vi "GUI_Tape_Alignment.vi"() -> ()   [LabVIEW 2020]
uses:
  Shared/GUI_Template/GUI_master/tcp_new_data_event.ctl
  Shared/GUI_Template/GUI_master/tcp new data cluster.ctl
  <vilib>/addons/_JKI.lib/Network_Streams_Connection.llb/NetworkCommand--Cluster.ctl
  <vilib>/addons/_JKI.lib/Network_Streams_Connection.llb/PublicSettings.ctl
  <vilib>/addons/_JKI.lib/Network_Streams_Connection.llb/NetworkConnection.lvclass/NetworkConnection.ctl
  <vilib>/Analysis/NI_AALPro.lvlib
  <vilib>/addons/_JKI.lib/Network_Streams_Connection.llb/NetworkConnection.lvclass
panel:
  out "ZCounts In Range?":bool=TRUE caption="Counts in range for\nz scan?"
  out "Max counts ok align":bool=TRUE
  in  "Min counts for align":dbl=200.0
  in  "Disable pointing correction":bool
  in  "+- from current":dbl=0.7 format="%#_13g"
  in  "set limits":bool caption="set limits basd on current position"
  in  "wangle upper limit":dbl=0.5682929999999999
  in  "wangle lower limit":dbl=-0.831707
  in  "vangle lower limit":dbl=-0.8982979999999999
  in  "vangle upper limit":dbl=0.501702
  out "move In Range W":bool=TRUE
  out "move In Range V":bool=TRUE
  in  "position::3":dbl=-3.999987 caption="vert stage pos" min=-48.0 max=0.0 step=0.01 format="%.5f"
  in  "GUIdevice 3":string="STAGE-PL1-Vertical"
  in  "Check beam quality":bool
  in  "Zpos Scan":bool
  in  "2ndmomW0y::1":dbl=55.508877 caption="w0 Y" min=0.0 max=999999.0
  in  "MaxCounts::1":dbl=1624.0 caption="Max Counts" min=0.0 max=999999999.0
  in  "xyzuvw::2":string="4.700098E+0,4.999902E+0,-1.803888E-7,1.749400E-6,-6.503994E-1,9.120211E-2" caption="Hex position"
  out "slow response":string="HEX-PL1-3-Small>>setxyzuvw>>4.700083,4.999904,0.000001,0.000007,-0.650383,0.091191>>no error,"
  in  "tab":T1(tab)=enum."Controls"
  out "Zpos and w0 Y":dbl(graph)=-4.0
  out "Alignment attempts":i32=3
  out "Waveform Chart 2":u32(graph)=298
  out "Movement time":u32=298
  out "Alignment time":u32=4006
  out "Waveform Chart 3":u32(graph)=4006
  out "Waveform Chart 4":i32(graph)=3
  out "Waveform Chart":cluster{"centroidx::1":dbl, "centroidy::1":dbl}(graph)={"centroidx::1"=1170.062134, "centroidy::1"=572.23645}
  out "Zpos and w0 Y 2":dbl(graph)=3261.0
  out "X Graph":T2(graph)
  out "Y Graph":T3(graph)
  out "X slope":dbl
  out "Y slope":dbl
  out "Y error":dbl
  out "X error":dbl
  in  "Calibration steps":dbl=8.0
  in  "Calibration Angle":cluster{"X":dbl, "Y":dbl}={"X"=0.01, "Y"=0.01}
  in  "Export":bool caption="Export calibration"
  in  "Import":bool caption="Import calibration"
  in  "Dont z scan if above this counts":dbl=2000.0
  in  "Central position of z scan":dbl=-4.0
  in  "Diagnostic type":enum16{"Max counts", "w0 Y"}(ring)
  in  "Disable Zpos Scan":bool=TRUE
  in  "zpos scan increment":dbl=1.0
  in  "zpos scan range":dbl=6.0
  in  "Newmark for vertical":bool=TRUE
  in  "Min counts for z scan":dbl=20.0
  in  "central z upper limit":dbl=-6.0
  in  "central z lower limit":dbl=-6.0
  in  "always z scan":bool
  in  "Buffer":dbl=0.9 format="%#_13g"
  in  "Accuracy limit":cluster{"X":dbl, "Y":dbl}={"X"=5.0, "Y"=5.0}
  out "Connected?":bool=TRUE
  in  "Aligned message":T4={"Command"="Alignment Done!", "Arguments"=variant(string "Arguments are variants. Wire anything!"), " Msg Id"=0}
  in  "Settings":T5={"My Name"="AlignmentGUI", "Remote IP Address"="", "Remote Name"="TapeDrive"}
  out "Public Settings":T5={"My Name"="AlignmentGUI", "Remote IP Address"="", "Remote Name"="TapeDrive"}
  out "Message count":i32=306
  out "Incoming Messages":T4[](array[typedef])=[{"Command"="ping", "Arguments"=variant, " Msg Id"=0}]
  out "Connected? 2":bool=TRUE
  in  "Stop z scan":bool
  out "Max vs z":T6(graph)={"Hexapod zscan positions"=[-9.0, -8.0, -7.0, -6.0, -5.0, -4.0, -3.0], "Hexapod zscan diagnostic"=[227.0, 362.0, 861.0, 1607.0, 1974.0, 3261.0, 1052.0]}
  out "msg":string="Macro: Alignment"
  out "tcp data event":T7
  in  "Target.Y::1":dbl=571.0 caption="Target Y" min=0.0 max=2000.0
  in  "Target.X::1":dbl=1173.0 caption="Target X" min=0.0 max=2000.0
  in  "Stop":bool
  out "Remaining States":string
  out "Current State":string="Exit"
  in  "Calibrate":bool
  in  "wangle::2":dbl=0.091202 caption="W" min=-1.0 max=1.0 step=0.01 format="%.5f"
  in  "vangle::2":dbl=-0.650399 caption="V" min=-1.0 max=1.0 step=0.01 format="%.5f"
  in  "centroidy::1":dbl=590.313232 caption="Centroid Y" min=0.0 max=0.0
  in  "centroidx::1":dbl=1182.786255 caption="Centroid X" min=0.0 max=0.0
  in  "ypos::2":dbl=4.999902 caption="Y" min=-10.0 max=10.0 step=0.01 format="%.5f"
  in  "xpos::2":dbl=4.700098 caption="X" min=-10.0 max=10.0 step=0.01 format="%.5f"
  in  "zpos::2":dbl=-0.0 caption="Z" min=-5.0 max=5.0 step=0.01 format="%.5f"
  in  "uangle::2":dbl=2e-06 caption="U" min=-1.0 max=1.0 step=0.01 format="%.5f"
  out "error IO 2":errorcluster
  in  "GUIdevice 2":string="HEX-PL1-3-Small"
  in  "GUIdevice 1":string="CAM-PL1-TapeDrivePointing"
  in  "Align Tape":bool
  # "Tape drive device cmd to align"
  # "Action: Get Beam Diagnostic>> Check Quality"
  # "disabled or counts high enough"
  # "If enabled. z scan only if max counts too low"
  # "Macro: Alignment"
  # "Macro: Hexapod Zpos Scan\nMacro: Alignment"
  # "Loop of\nAction: Move>> Zpos Scan\nAction: Get Beam Diagnostic>>Zpos Scan\n\nThen \n\nAction: Find Best Zpos"
  # "Align Tape button"
  # "Macro: Alignment"
  # "Action: Find Best Zpos\n#which calls\nAction: Move>> Best Zpos\nMacro: Alignment\n#does aligment get called twice?"
  # "Counts too low or disabled"
  # "If enabled and sufficient counts"
  # "Do nothing"
  # "Update: Alignment Constants\nAction: Get Centroid>> Align"
  # "If aligned or  align disabled"
  # "Action: Move>> Align\nAction: Get Centroid>> Align"
  # "Action: Send Response"
  # "Note: If action move tries too many times, it empties state machine and tape drive never gets a response"
  # "Align"
  # "Z scan"
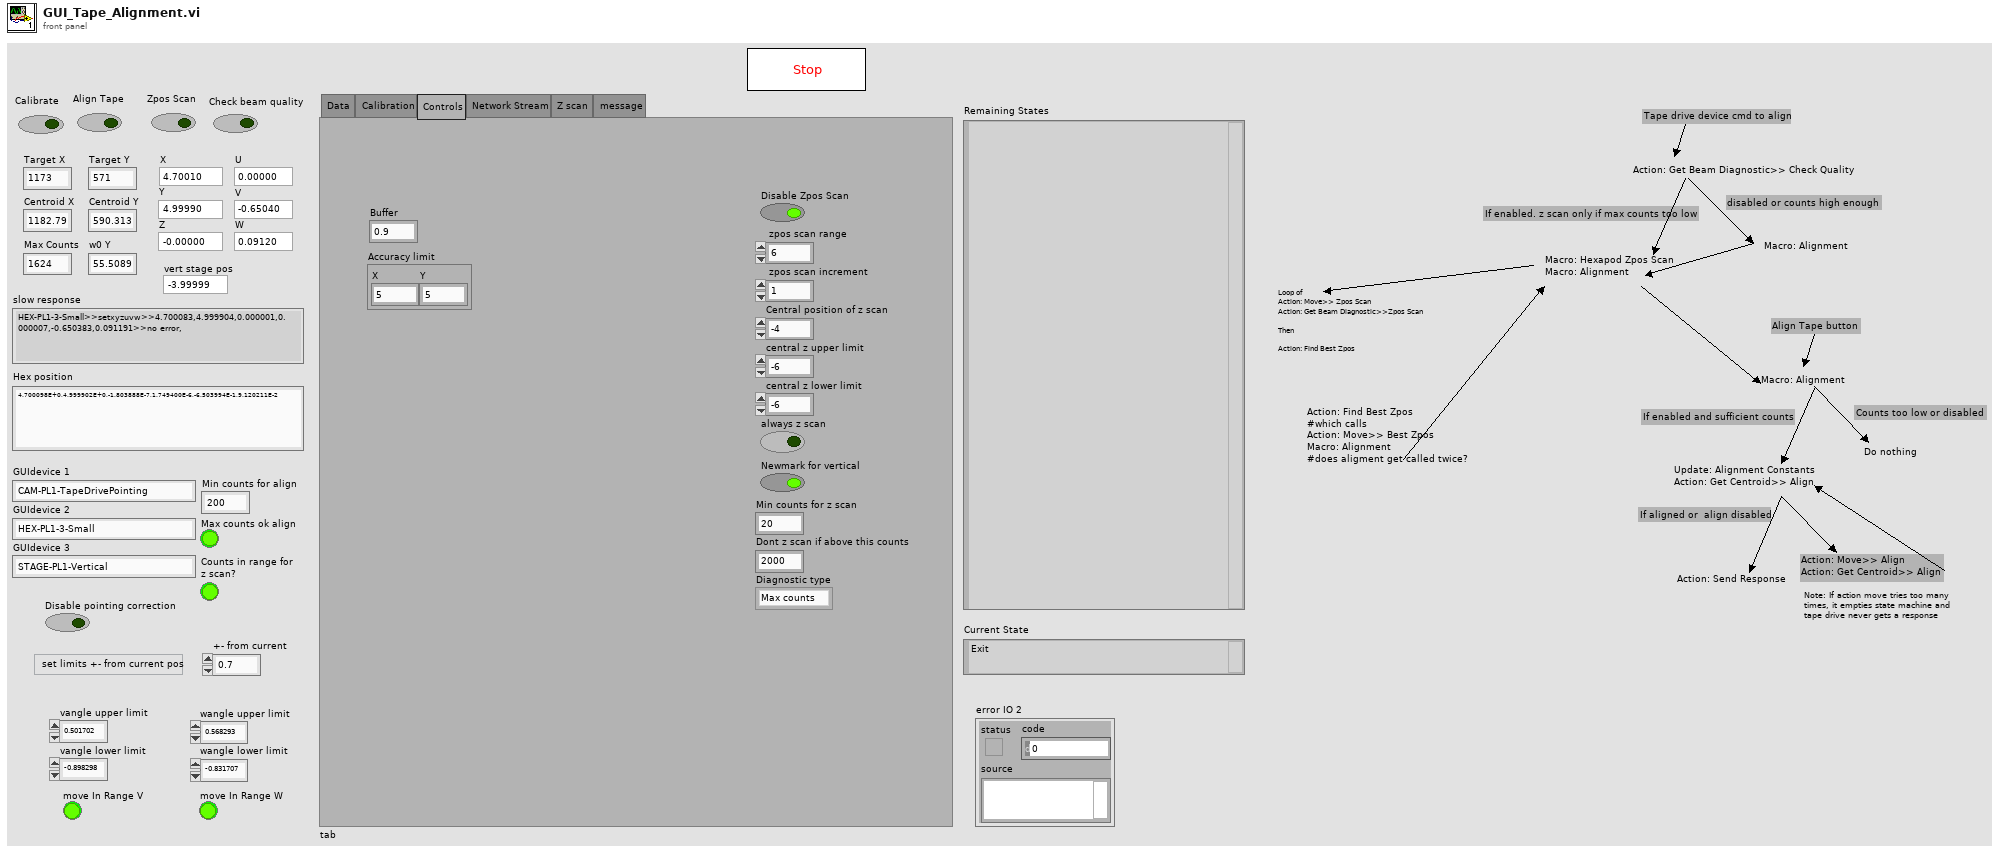
[diagram p1: front panel]
types:
  T1 = enum32{"Data", "Calibration", "Controls", "Network Stream", "Z scan", "message"}
  T2 = cluster{"Centroids.x":dbl[], "Best Linear Fit":dbl[]}[]
  T3 = cluster{"Centroids.y":dbl[], "Best Linear Fit":dbl[]}[]
  T4 = typedef "NetworkConnection.lvclass/NetworkCommand--Cluster.ctl" = cluster{"Command":string, "Arguments":variant, " Msg Id":i32}
  T5 = typedef "NetworkConnection.lvclass/PublicSettings.ctl" = cluster{"My Name":string, "Remote IP Address":string, "Remote Name":string}
  T6 = cluster{"Hexapod zscan positions":dbl[], "Hexapod zscan diagnostic":dbl[]}
  T7 = typedef "tcp_new_data_event.ctl" = refnum<user-event>
  T8 = typedef "tcp new data cluster.ctl" = cluster{"EventEnum":enum16{"new data", "connection status update"}, "Device name":string}
  T9 = enum32{"Data", "Calibration", "Controls", "Network Stream", "Z scan"}
  T10 = enum32{"Invalid", "Standard", "Closed", "Hidden", "Minimized", "Maximized"}
  T11 = enum32{"invalid app kind", "Development System", "Run Time System", "Student Edition", "Embedded LabVIEW", "Evaluation", "Custom"}
  T12 = cluster{"Messages[0]":T4, "Messages[1]":T4, "Messages[2]":T4, "Messages[3]":T4, "Messages[4]":T4, "Messages[5]":T4, "Messages[6]":T4, "Messages[7]":T4, "Messages[8]":T4}
  T13 = cluster{"Core":cluster{"Current VI Reference":refnum<vi>, "Close Panel on Exit?":bool}, "Difference":cluster{"X":dbl, "Y":dbl}, "Scale Factor":cluster{"X":dbl, "Y":dbl}, "Centroids":cluster{"Centroids.x":dbl[], "Centroids.y":dbl[]}, "Calibration Angle ":cluster{"X":dbl, "Y":dbl}, "Accuracy limit":cluster{"X":dbl, "Y":dbl}, "Calibration steps":dbl, "NetworkConnection out":refnum<class "NetworkConnection.lvclass">, "Messages":i32, "Alignment attempts":i32, "Timer":cluster{"T1":i32, "T2":i32}, "Hexapod positions":cluster{"P1":string, "P2":string}, "Beam diagnostic cutoffs":cluster{"MaxCounts":dbl, "w0 Y":dbl}, "Hexapod zscan data":cluster{"Hexapod zscan positions":dbl[], "Hexapod zscan diagnostic":dbl[], "Index":i32, "Best Zpos":dbl}, "Diagnostic type":string}
  T14 = cluster{"Hexapod zscan positions":dbl[], "Hexapod zscan diagnostic":dbl[], "Index":i32, "Best Zpos":dbl}
  T15 = cluster{"Centroids.x":dbl[], "Centroids.y":dbl[]}
  T16 = cluster{"Current VI Reference":refnum<vi>, "Close Panel on Exit?":bool}
  T17 = cluster{"Centroids.x":dbl[], "Best Linear Fit":dbl[]}
  T18 = cluster{"Centroids.y":dbl[], "Best Linear Fit":dbl[]}
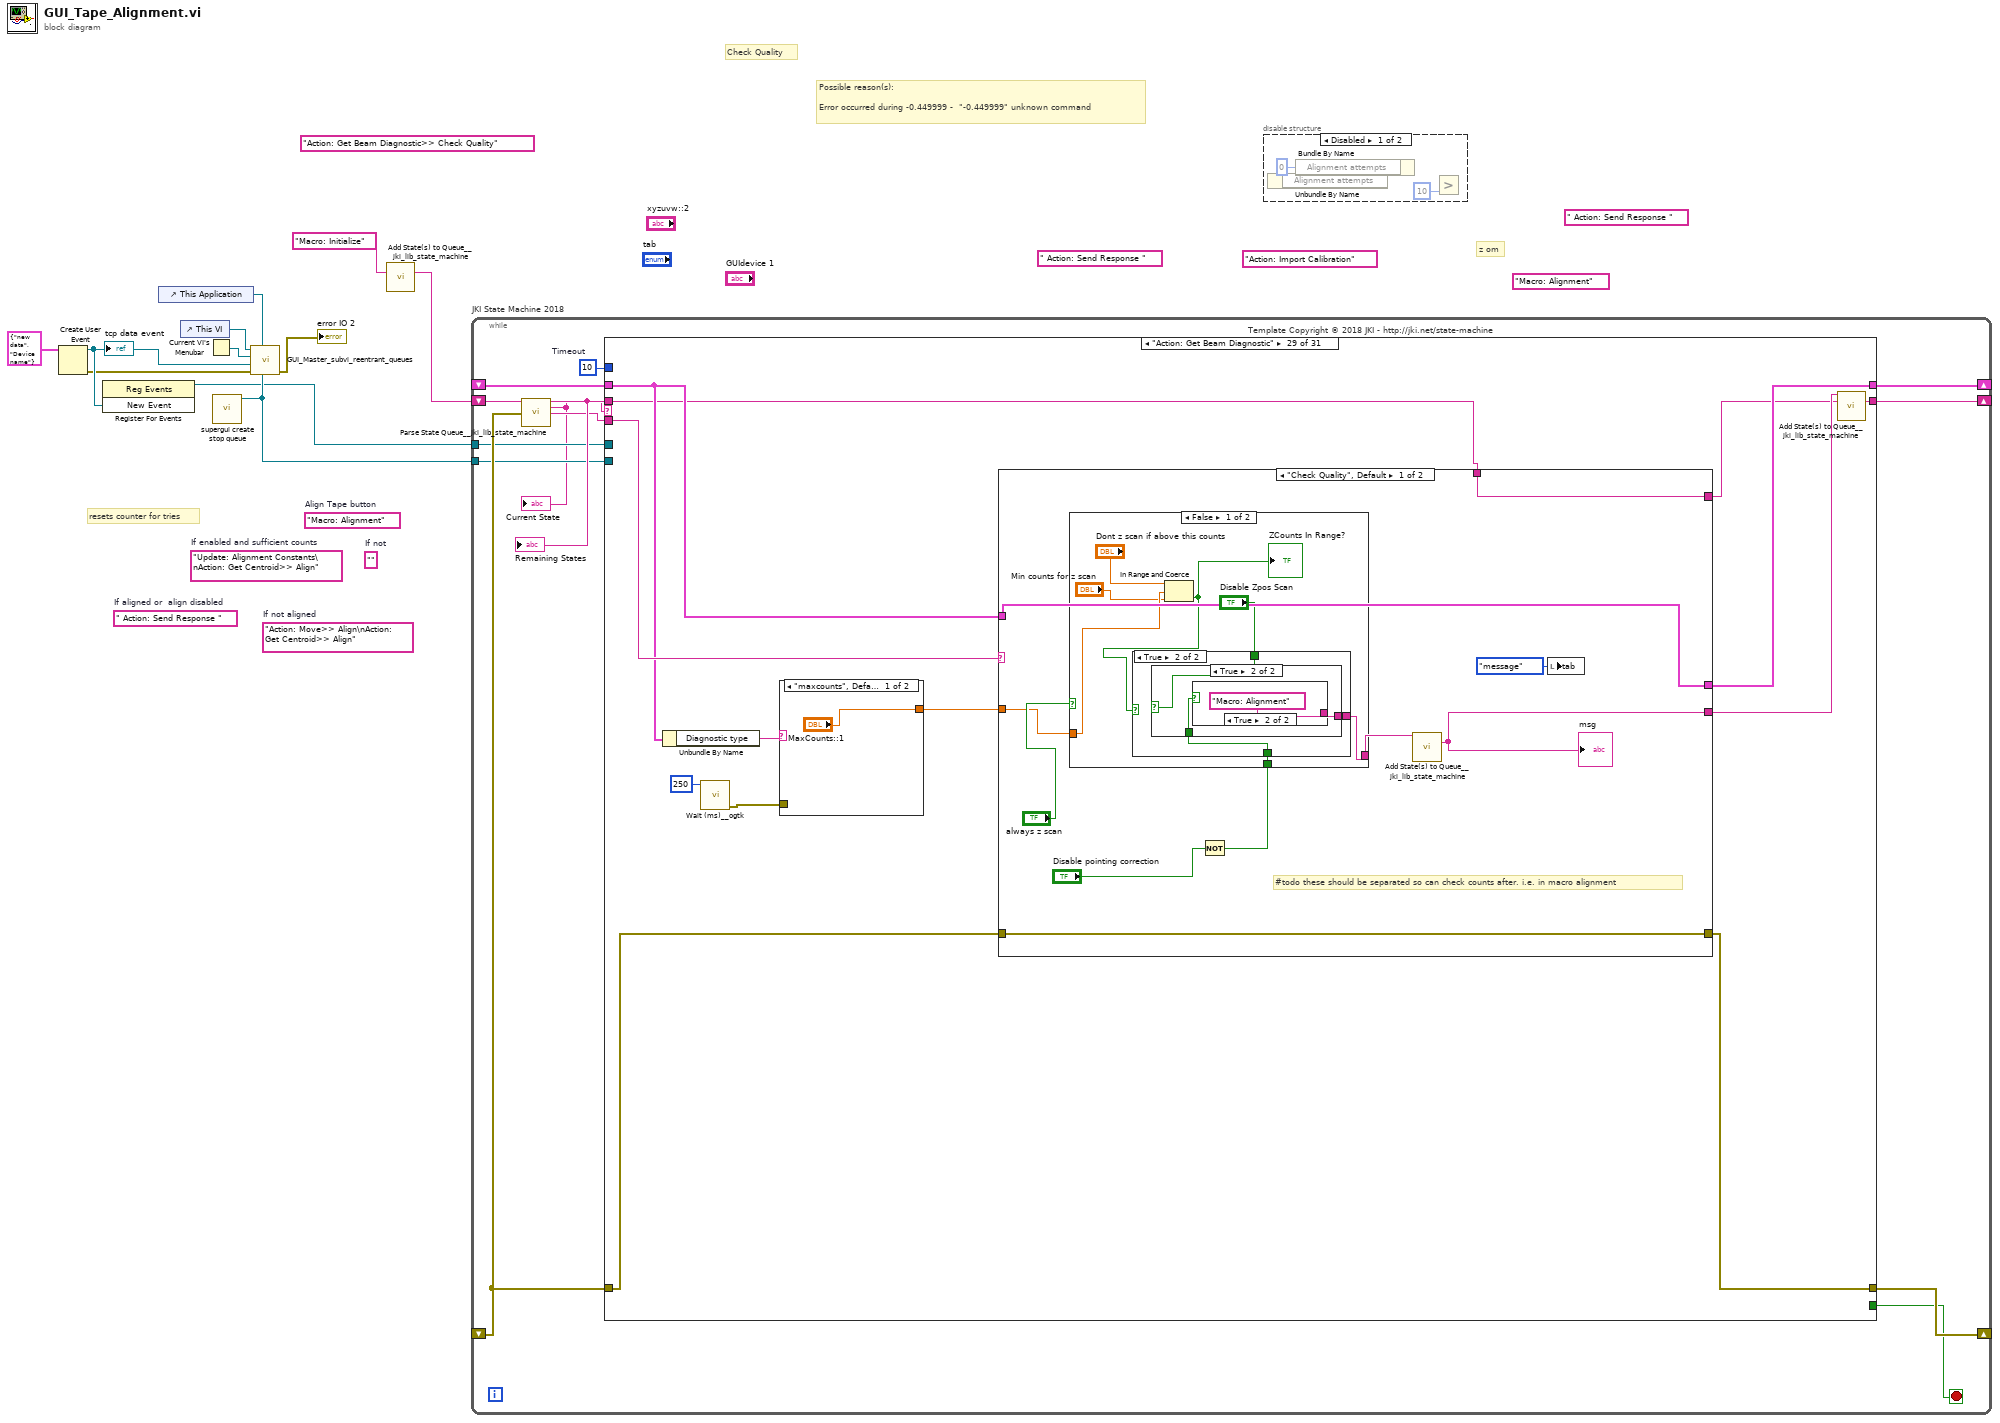
[diagram p0: block diagram]
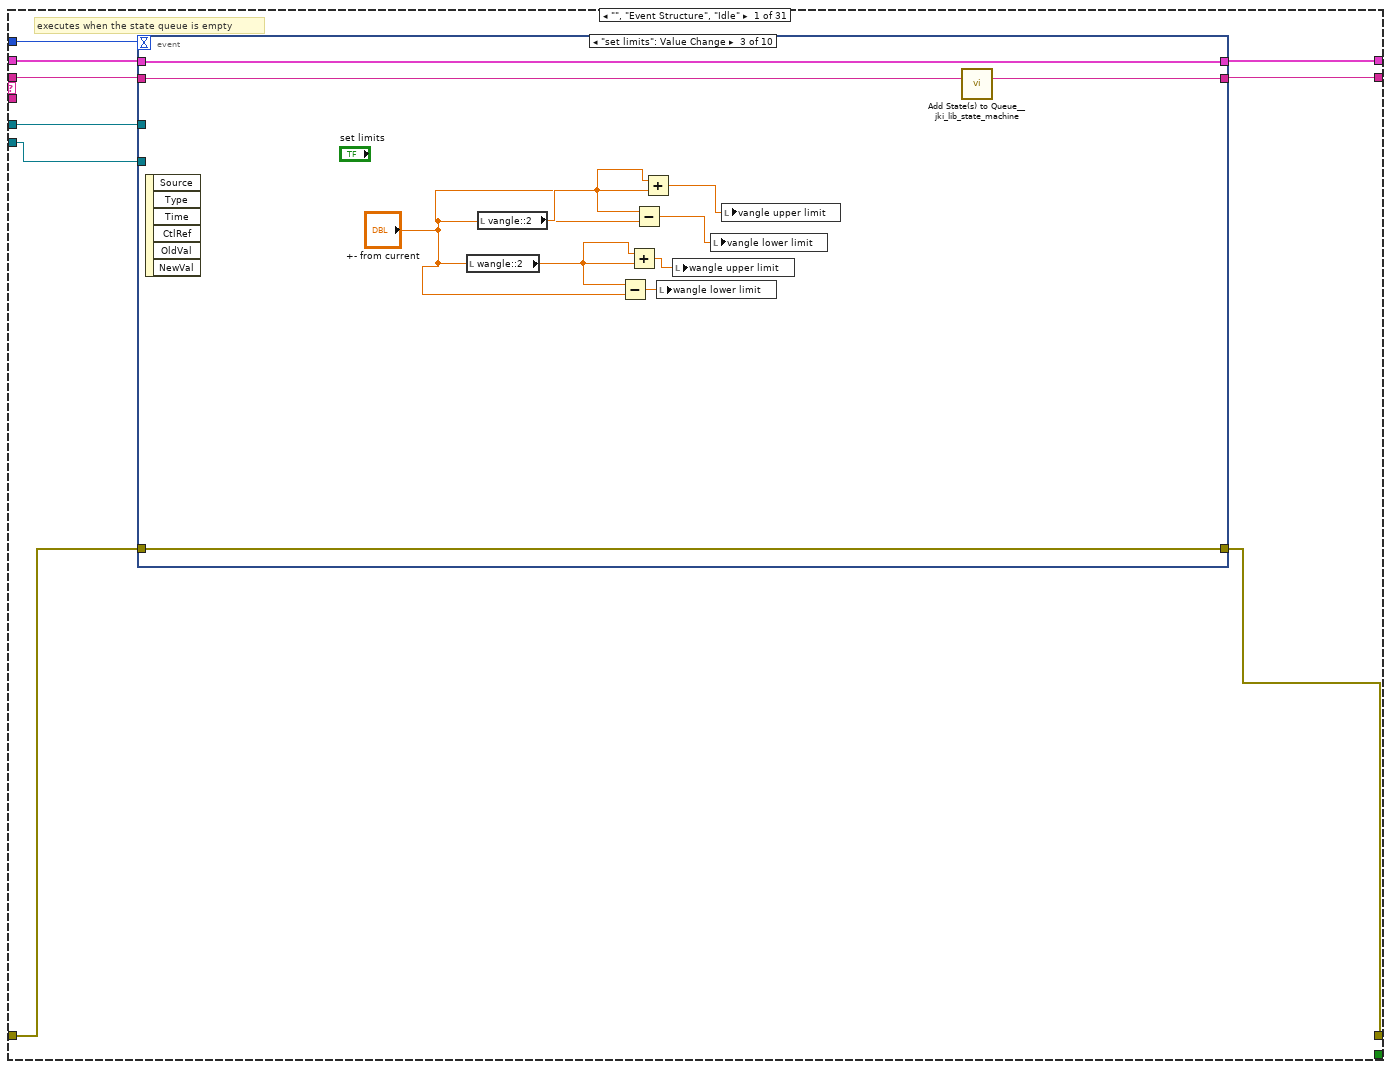
[diagram p3: hidden frame]
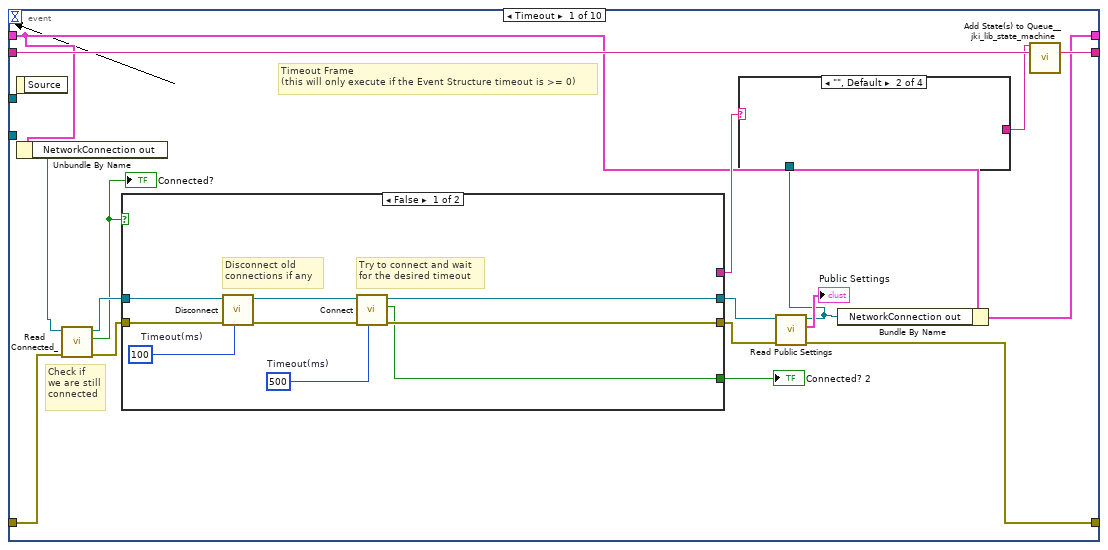
[diagram p4: hidden frame]
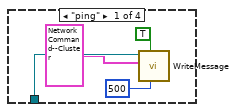
[diagram p5: hidden frame]
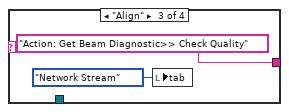
[diagram p6: hidden frame]
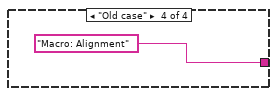
[diagram p7: hidden frame]
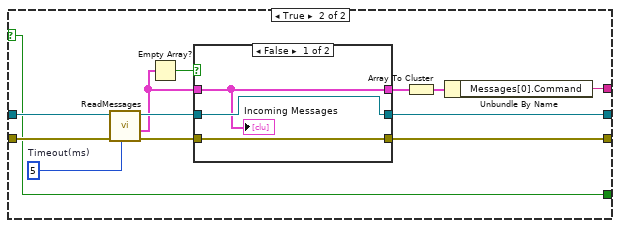
[diagram p8: hidden frame]
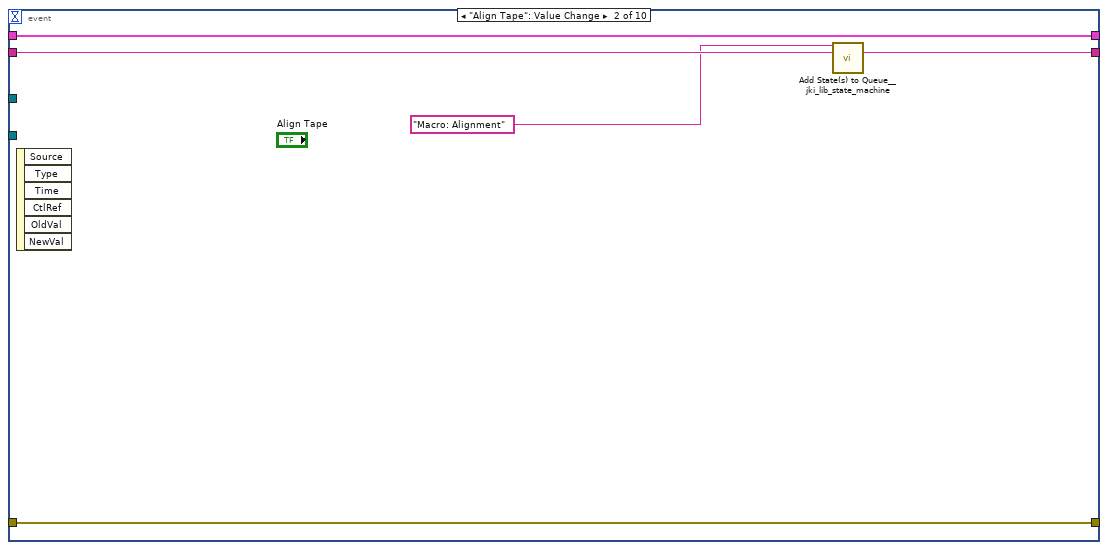
[diagram p10: hidden frame]
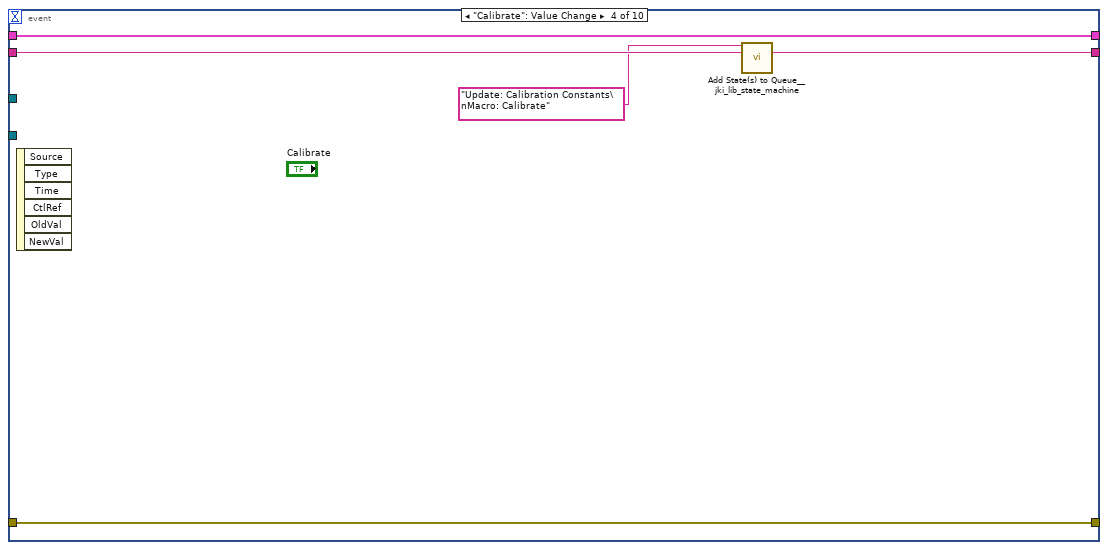
[diagram p11: hidden frame]
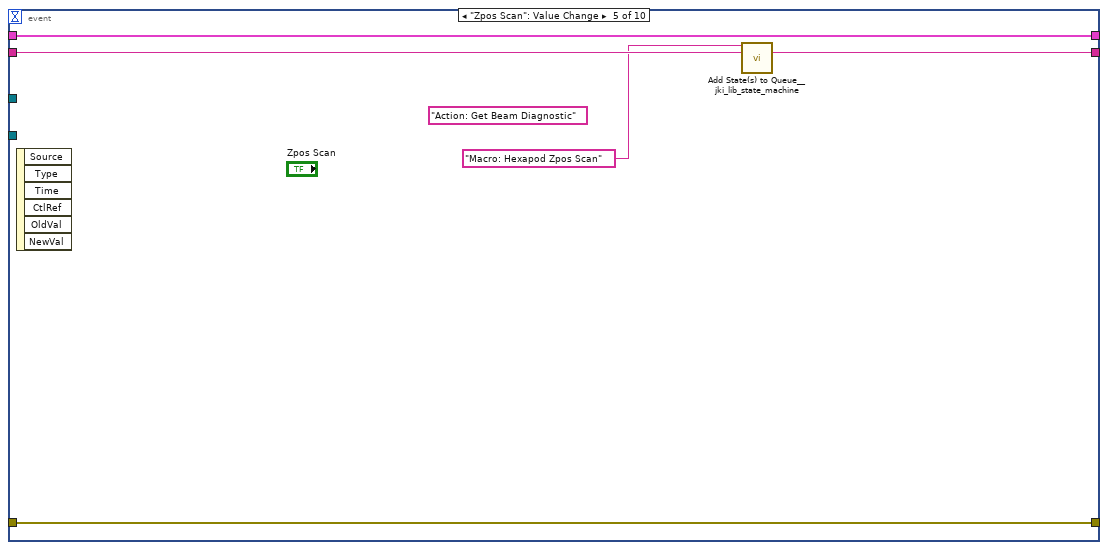
[diagram p12: hidden frame]
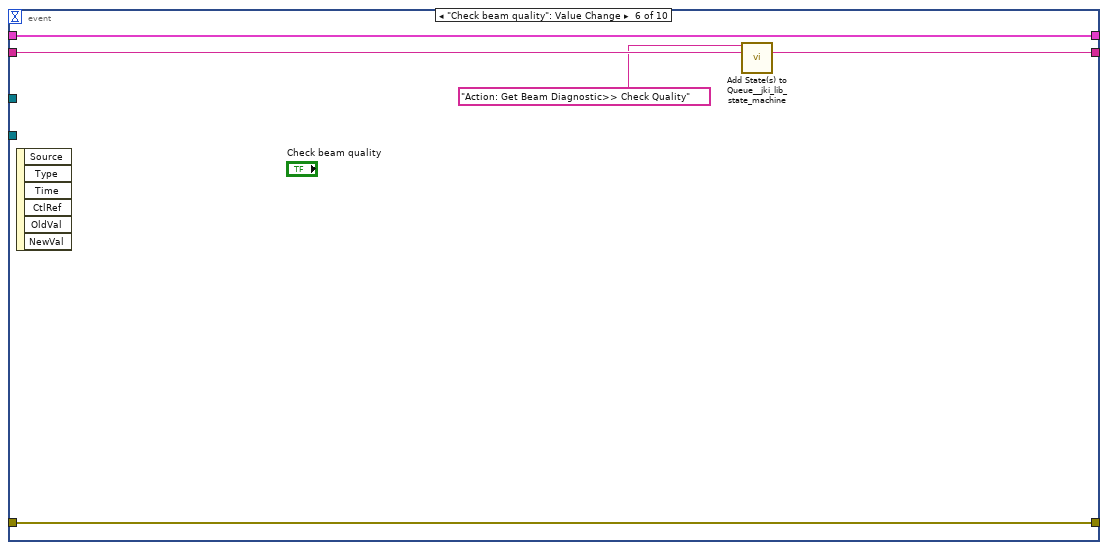
[diagram p13: hidden frame]
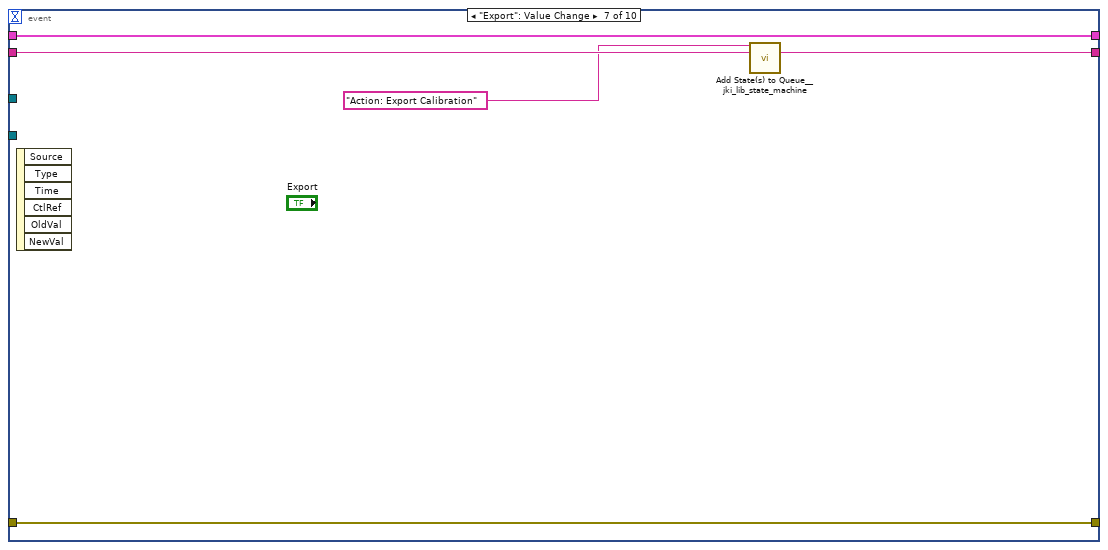
[diagram p14: hidden frame]
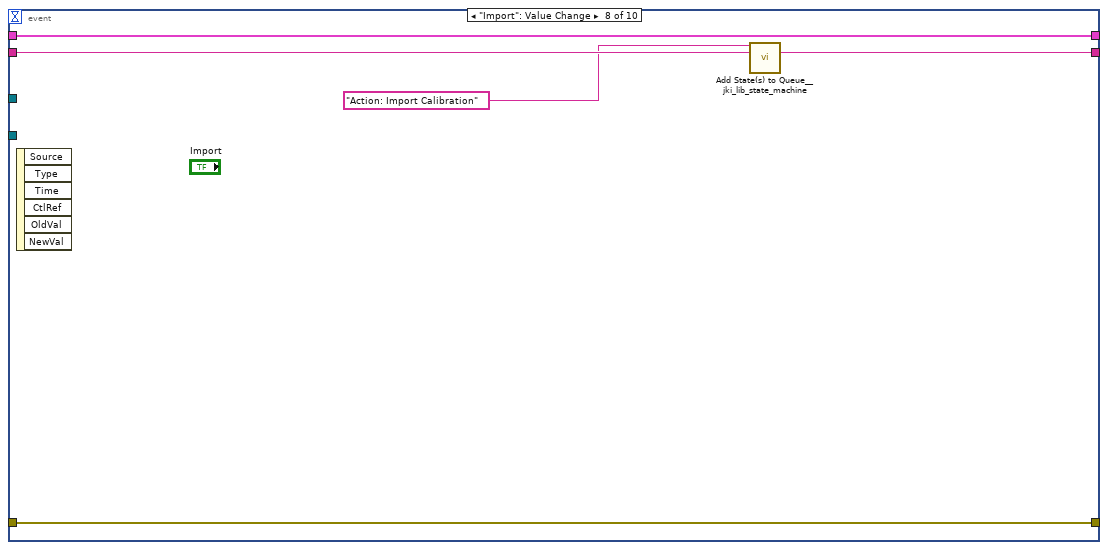
[diagram p15: hidden frame]
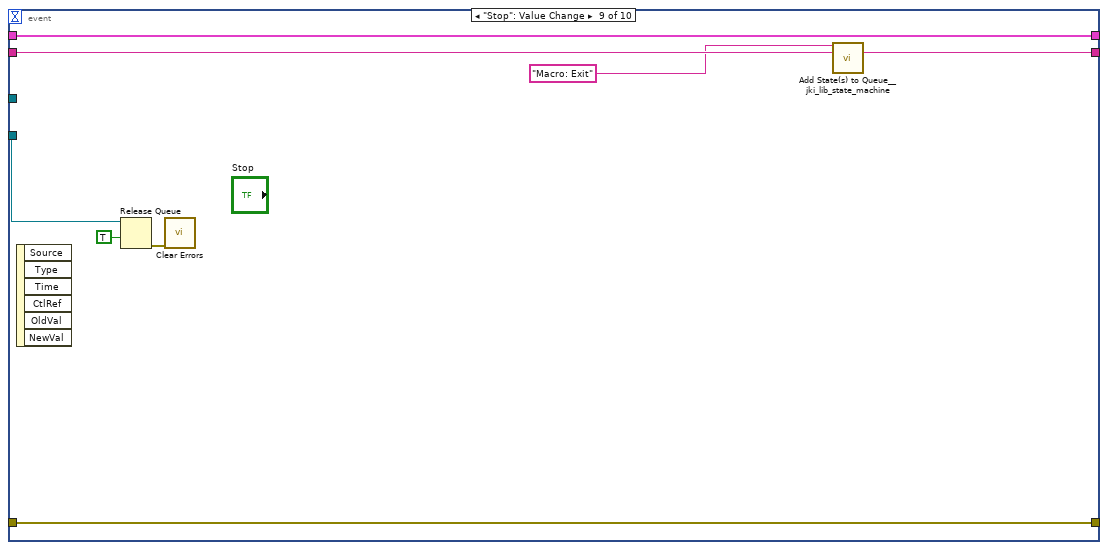
[diagram p16: hidden frame]
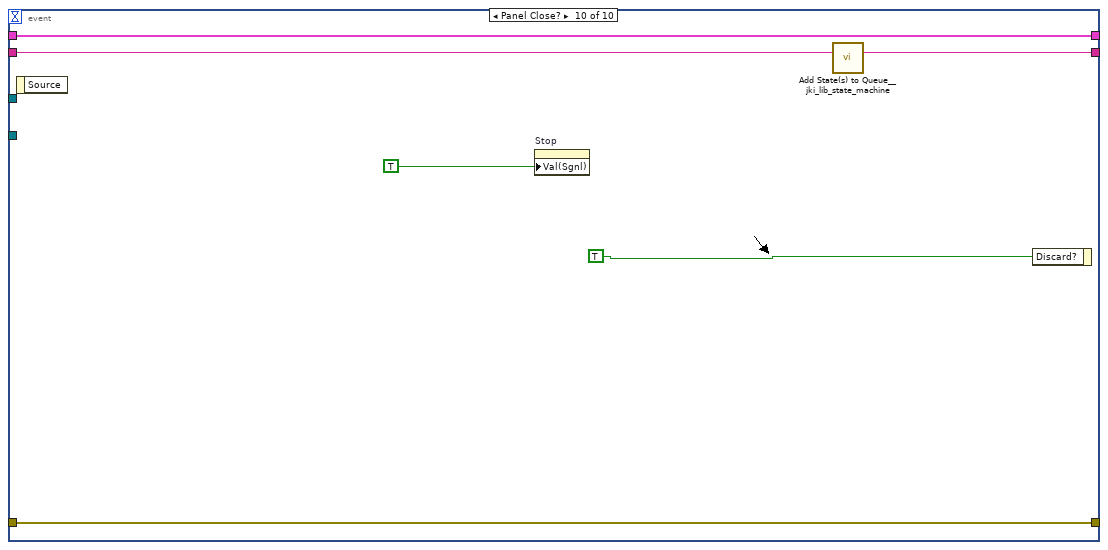
[diagram p17: hidden frame]
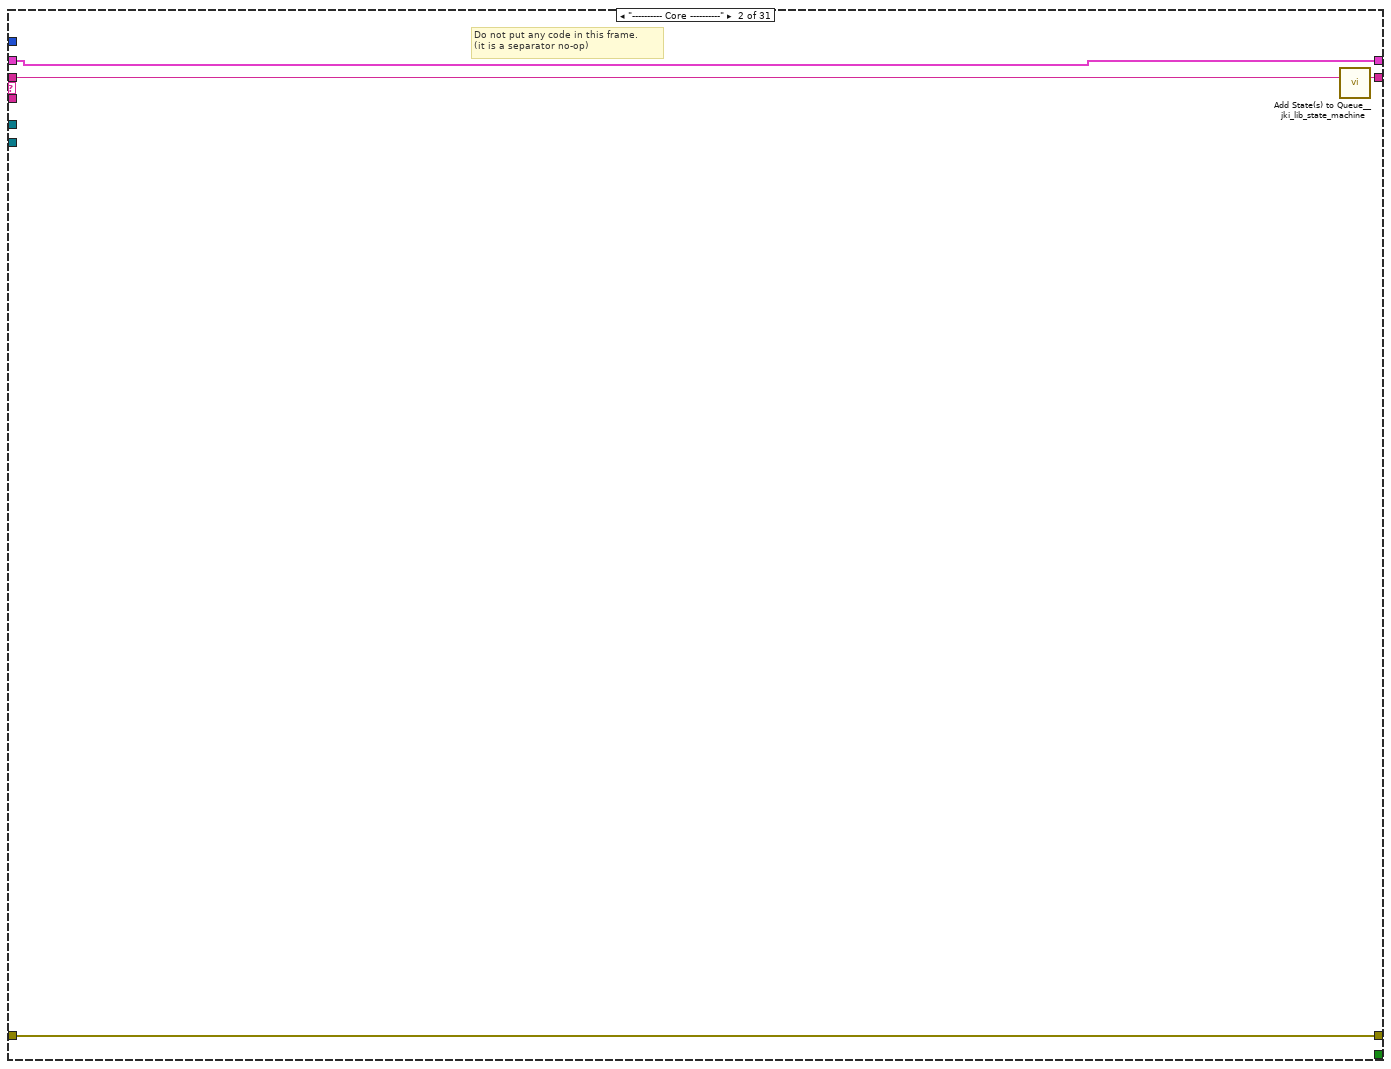
[diagram p18: hidden frame]
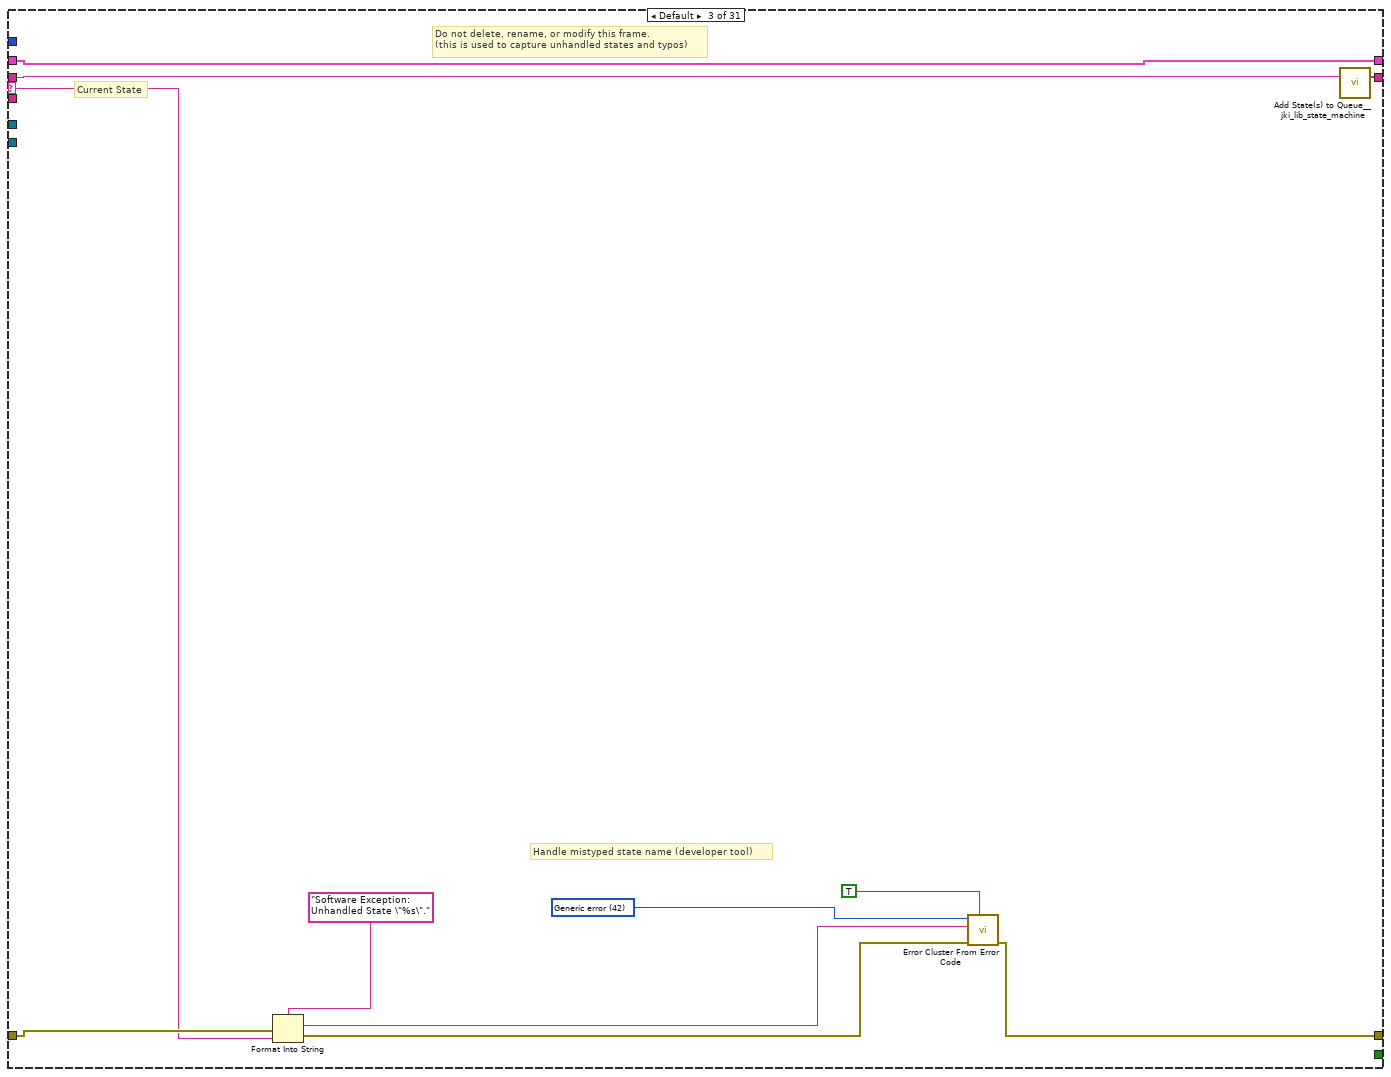
[diagram p19: hidden frame]
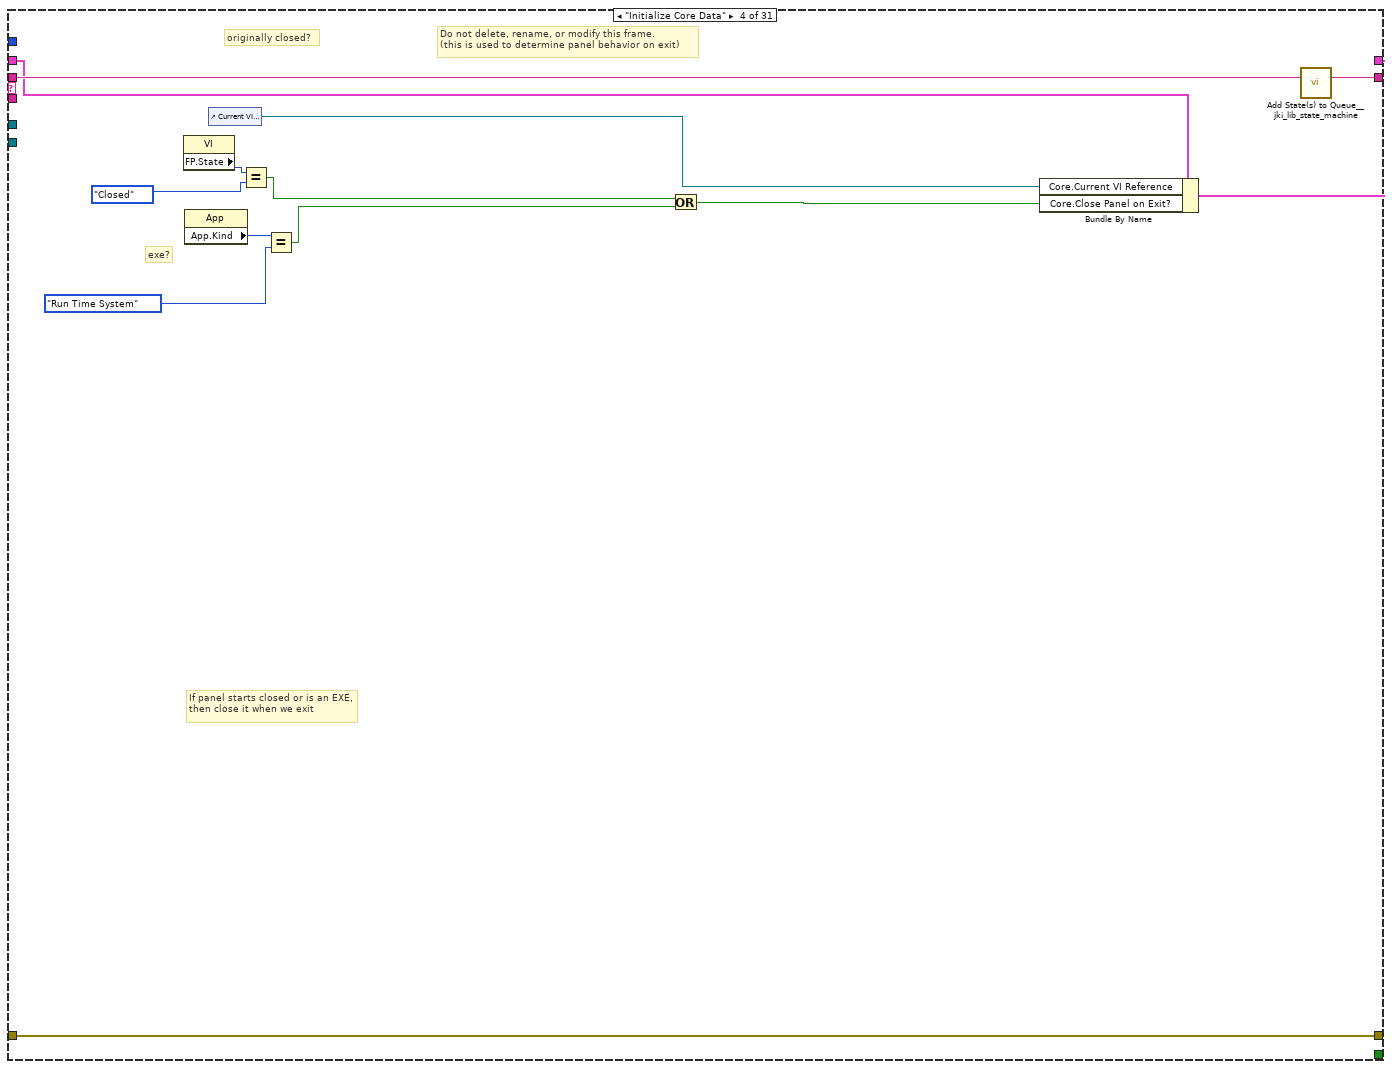
[diagram p20: hidden frame]
diagram:
  (unwired) " Action: Send Response "
  (unwired) "Action: Get Beam Diagnostic>> Check Quality"
  (unwired) "Action: Move>> Align\nAction: Get Centroid>> Align"  # If not aligned
  (unwired) " Action: Send Response "  # If aligned or  align disabled
  (unwired) ""  # If not
  (unwired) "Update: Alignment Constants\nAction: Get Centroid>> Align"  # If enabled and sufficient counts
  (unwired) "Macro: Alignment"  # Align Tape button
  (unwired) " Action: Send Response "
  (unwired) "Action: Import Calibration"
  (unwired) "Macro: Alignment"
  # "resets counter for tries"
  # "z om"
  # "Check Quality"
  # "Possible reason(s):\n\nError occurred during -0.449999 -  \"-0.449999\" unknown command"
  n1 = Create User Event(user event datatype=T8 {"EventEnum"=enum."new data", "Device name"="Device name"} ("New Event")) -> (user event=w8:refnum<user-event>, error out=w7:errorcluster)  [unwired: 1 in]
  "tcp data event" <- w8
  n2 = register-events(w8) -> (reference out=w1:refnum<event-registration>)  [unwired: 2 in, 1 out]
  n3 = control-ref of="This Application"() -> (w9:refnum<vi>)
  n4 = control-ref of="This VI"() -> (w4:refnum<vi>)
  n5 = Current VI's Menubar() -> (w5:refnum<k9>)
  n6 = call "supergui create stop queue.vi"() -> ("STOP Queue out"=w2:refnum<queue>)  [unwired: 11 in]
  n7 = call "GUI_Master_subvi_reentrant_queues.vi"("STOP Queue in"=w2, "This Application"=w9, "error in (no error)"=w7, "tcp data event"=w8, "Caller menu reference"=w5, "Caller VI ref"=w4) -> ("error out"=→"error IO 2":errorcluster)  [unwired: 5 in]
  n8 = call <vilib>:"Add State(s) to Queue__jki_lib_state_machine.vi"("State(s) in (\"\")"="Macro: Initialize") -> ("States Out"=w11:string)  [unwired: 14 in]
  n9 = while "JKI State Machine 2018" {
    shift-right: [w19] -> _
    shift-left: _ -> [w18]
    shift-right: [w21] -> _
    shift-left: _ -> [w16]
    shift-right: [w20] -> _
    shift-left: w11 -> [w22]
    tunnel: w1 -> [w15]
    tunnel: w2 -> [w14]
    stop <- w13 stop-if-true
    w17 = 10  # Timeout
    # "Template Copyright © 2018 JKI - http://jki.net/state-machine"
    n10 = call <vilib>:"Parse State Queue__jki_lib_state_machine.vi"("State Queue"=w22, "Error In (no error)"=w16) -> ("Remaining States"=w24:string, "Current State"=w12:string, "Arguments"=w23:string)  [unwired: 11 in]
    "Current State" <- w12
    "Remaining States" <- w24
    n11 = case shown="\"Action: Get Beam Diagnostic\"" w12 {
      selector: w12 -> [_ _ w145 _ _ _ _ _ _ _ _ _ _ _ _ _ _ _ _ _ _ _ _ _ _ _ _ _ _ _ _]
      tunnel: w24 -> [w33 w144 w149 w168 w174 w179 w183 w203 w211 w215 w219 w225 w236 w305 w310 w320 w339 w372 w394 w401 w407 w415 w420 w434 w477 w659 w667 w678 w680 w755 w779]
      tunnel: w23 -> [_ _ _ _ _ _ _ _ _ _ _ w220 w230 _ _ _ _ _ _ _ _ _ _ w424 w476 _ _ _ w690 _ _]
      tunnel: w18 -> [w31 w141 w147 w161 w171 w177 w180 _ w207 w212 w217 w223 w232 w302 w307 w313 w343 w368 w391 w398 w405 w414 w417 w425 w502 w655 w665 w673 w684 w752 w772]
      tunnel: [w30 w142 w151 w165 errorcluster {"status"=FALSE, "code"=0, "source"=""} ("error out") w176 w181 w200 w204 w213 w216 w221 w233 w303 w308 w322 w351 w373 w392 w399 w408 w410 w418 w426 w495 w657 w661 w668 w685 w753 w766] -> w21
      tunnel: w16 -> [w29 w142 w150 w165 w170 w176 w181 w200 w208 w213 w216 w222 w234 w303 w308 w322 w351 w373 w392 w399 w408 w410 w418 w423 w501 w657 w662 w669 w686 w753 w776]
      tunnel: [w32 w143 w148 w167 w173 w178 w182 w202 w210 w214 w218 w224 w235 w304 w309 w323 w352 w374 w393 w400 w409 w416 w419 w433 w503 w658 w666 w677 w691 w754 w778] -> w20
      tunnel: [_ _ _ _ _ TRUE _ _ _ _ _ _ _ _ _ _ _ _ _ _ _ _ _ _ _ _ _ _ _ _ _] -> w13
      tunnel: [w28 w141 w147 w166 w171 w177 w180 w201 w207 w212 w217 w223 w232 w302 w307 w311 w342 w369 w391 w398 w404 w413 w417 w432 w481 w656 w665 w676 w687 w751 w773] -> w19
      tunnel: w17 -> [w27 _ _ _ _ _ _ _ _ _ _ _ _ _ _ _ _ _ _ _ _ _ _ _ _ _ _ _ _ _ _]
      tunnel: w15 -> [w26 _ _ _ _ _ _ _ _ _ _ _ _ _ _ _ _ _ _ _ _ _ _ _ _ _ _ _ _ _ _]
      tunnel: w14 -> [w25 _ _ _ _ _ _ _ _ _ _ _ _ _ _ _ _ _ _ _ _ _ _ _ _ _ _ _ _ _ _]
      frame "", "Event Structure", "Idle" {
        # "executes when the state queue is empty"
        n12 = event shown="[2] \"set limits\": Value Change" {
          selector: _ -> [_ _ _ _ _ _ _ _ _ _]
          dyn-events: _ -> [_ _ _ _ _ _ _ _ _ _]
          timeout: w27 -> [_ _ _ _ _ _ _ _ _ _]
          tunnel: w33 -> [w50 w90 w101 w105 w110 w115 w119 w124 w134 w140]
          tunnel: [w49 w89 w100 w103 w109 w113 w120 w125 w133 w139] -> w32
          tunnel: w31 -> [w40 w86 w98 w106 w111 w116 w121 w126 w131 w137]
          tunnel: [w37 w88 w99 w102 w108 w112 w117 w122 w132 w138] -> w30
          tunnel: w29 -> [w45 w88 w99 w102 w108 w112 w117 w122 w132 w138]
          tunnel: [w41 w86 w98 w106 w111 w116 w121 w126 w131 w137] -> w28
          tunnel: w26 -> [_ _ _ _ _ _ _ _ _ _]
          tunnel: w25 -> [_ _ _ _ _ _ _ _ w127 _]
          event Timeout {
            # "Check if\nwe are still\nconnected"
            # "Timeout Frame\n(this will only execute if the Event Structure timeout is >= 0)"
            n13 = event-data() -> ()  [unwired: 1 in, 1 out]
            n14 = Unbundle By Name(w40) -> ("NetworkConnection out"=w42:refnum<class "NetworkConnection.lvclass">)
            n15 = call <vilib>:"Read Connected_.vi"("error in (no error)"=w45, "NetworkConnection in"=w42) -> ("error out"=w48:errorcluster, "Connected?"=w46:bool, "NetworkConnection out"=w47:refnum<class "NetworkConnection.lvclass">)  [unwired: 7 in]
            "Connected?" <- w46
            n16 = case shown="False" w46 {
              selector: w46 -> [_ w67]
              tunnel: w48 -> [w62 w77]
              tunnel: w47 -> [w64 w78]
              tunnel: [w65 w72] -> w39
              tunnel: [w66 w71] -> w38
              tunnel: [_ w75] -> w44
              tunnel: [w58 w67] -> w35
              frame False {
                w59 = 500  # Timeout(ms)
                w60 = 100  # Timeout(ms)
                # "Try to connect and wait\nfor the desired timeout"
                # "Disconnect old\nconnections if any"
                n17 = call <vilib>:"Disconnect.vi"("Timeout ms (1000)"=w60, "error in (no error)"=w62, "NetworkConnection in"=w64) -> ("error out"=w61:errorcluster, "NetworkConnection out"=w63:refnum<class "NetworkConnection.lvclass">)  [unwired: 7 in]
                n18 = call <vilib>:"Connect.vi"("Timeout(ms)"=w59, "error in (no error)"=w61, "NetworkConnection in"=w63) -> ("error out"=w66:errorcluster, "Connected?"=w58:bool, "NetworkConnection out"=w65:refnum<class "NetworkConnection.lvclass">)  [unwired: 6 in]
              }
              frame True {
                w79 = 5  # Timeout(ms)
                n19 = call <vilib>:"ReadMessages.vi"("Timeout(ms)"=w79, "error in (no error)"=w77, "NetworkConnection in"=w78) -> ("error out"=w70:errorcluster, "Messages"=w68:T4[], "NetworkConnection out"=w73:refnum<class "NetworkConnection.lvclass">)  [unwired: 4 in, 2 out]
                n20 = Empty Array?(array=w68) -> (empty?=w74:bool)
                n21 = case shown="False" w74 {
                  tunnel: w73 -> [w82 w85]
                  tunnel: [w82 w85] -> w72
                  tunnel: [w81 w84] -> w71
                  tunnel: w70 -> [w81 w84]
                  tunnel: [w80 w83] -> w69
                  tunnel: w68 -> [w80 w83]
                  frame False {
                    "Incoming Messages" <- w80
                  }
                  frame True {
                  }
                }
                n22 = Array To Cluster(array=w69) -> (cluster=w76:T12)
                n23 = Unbundle By Name(w76) -> ("Messages[0].Command"=w75:string)
              }
            }
            "Connected? 2" <- w35
            n24 = call <vilib>:"Read Public Settings.vi"("error in (no error)"=w38, "NetworkConnection in"=w39) -> ("error out"=w37:errorcluster, "Public Settings"=→"Public Settings":T5, "NetworkConnection out"=w34:refnum<class "NetworkConnection.lvclass">)  [unwired: 7 in]
            n25 = case shown="\"\", Default" w44 {
              tunnel: [_ _ "Action: Get Beam Diagnostic>> Check Quality" "Macro: Alignment"] -> w43
              tunnel: w34 -> [w54 _ _ _]
              frame "ping" {
                n26 = call <vilib>:"WriteMessage.vi"("Timeout(ms)"=500, "Wait for Ack? (false)"=TRUE, "Message"=T4 {"Command"="ping", "Arguments"=variant, " Msg Id"=-1}, "NetworkConnection in"=w54) -> ()  [unwired: 4 in, 4 out]
              }
              frame "", Default {
              }
              frame "Align" {
                n27 = local write "tab"(T9."Network Stream" ("tab")) -> ()
              }
              frame "Old case" {
              }
            }
            n28 = Bundle By Name(cluster=w40, "NetworkConnection out"=w34) -> (w41:T13)
            n29 = call <vilib>:"Add State(s) to Queue__jki_lib_state_machine.vi"("State(s) in Front (\"\")"=w43, "State(s) in (\"\")"=w50) -> ("States Out"=w49:string)  [unwired: 13 in]
          }
          event "Align Tape": Value Change {
            n30 = event-data() -> ()  [unwired: 1 in, 6 out]
            n31 = call <vilib>:"Add State(s) to Queue__jki_lib_state_machine.vi"("State(s) in Front (\"\")"="Macro: Alignment", "State(s) in (\"\")"=w90) -> ("States Out"=w89:string)  [unwired: 13 in]
          }
          event "set limits": Value Change {
            n32 = event-data() -> ()  [unwired: 1 in, 6 out]
            n33 = local read "wangle::2"() -> (w95:dbl)
            n34 = local read "vangle::2"() -> (w92:dbl)
            n35 = Subtract(x=w95, y="+- from current") -> (x-y=w97:dbl)
            n36 = Add(x=w95, y="+- from current") -> (x+y=w96:dbl)
            n37 = Subtract(x=w92, y="+- from current") -> (x-y=w94:dbl)
            n38 = Add(x=w92, y="+- from current") -> (x+y=w93:dbl)
            n39 = local write "wangle lower limit"(w97) -> ()
            n40 = local write "wangle upper limit"(w96) -> ()
            n41 = local write "vangle lower limit"(w94) -> ()
            n42 = local write "vangle upper limit"(w93) -> ()
            n43 = call <vilib>:"Add State(s) to Queue__jki_lib_state_machine.vi"("State(s) in (\"\")"=w101) -> ("States Out"=w100:string)  [unwired: 14 in]
          }
          event "Calibrate": Value Change {
            n44 = event-data() -> ()  [unwired: 1 in, 6 out]
            n45 = call <vilib>:"Add State(s) to Queue__jki_lib_state_machine.vi"("State(s) in Front (\"\")"="Update: Calibration Constants\nMacro: Calibrate", "State(s) in (\"\")"=w105) -> ("States Out"=w103:string)  [unwired: 13 in]
          }
          event "Zpos Scan": Value Change {
            (unwired) "Action: Get Beam Diagnostic"
            n46 = event-data() -> ()  [unwired: 1 in, 6 out]
            n47 = call <vilib>:"Add State(s) to Queue__jki_lib_state_machine.vi"("State(s) in Front (\"\")"="Macro: Hexapod Zpos Scan", "State(s) in (\"\")"=w110) -> ("States Out"=w109:string)  [unwired: 13 in]
          }
          event "Check beam quality": Value Change {
            n48 = event-data() -> ()  [unwired: 1 in, 6 out]
            n49 = call <vilib>:"Add State(s) to Queue__jki_lib_state_machine.vi"("State(s) in Front (\"\")"="Action: Get Beam Diagnostic>> Check Quality", "State(s) in (\"\")"=w115) -> ("States Out"=w113:string)  [unwired: 13 in]
          }
          event "Export": Value Change {
            n50 = event-data() -> ()  [unwired: 1 in, 6 out]
            n51 = call <vilib>:"Add State(s) to Queue__jki_lib_state_machine.vi"("State(s) in Front (\"\")"="Action: Export Calibration", "State(s) in (\"\")"=w119) -> ("States Out"=w120:string)  [unwired: 13 in]
          }
          event "Import": Value Change {
            n52 = event-data() -> ()  [unwired: 1 in, 6 out]
            n53 = call <vilib>:"Add State(s) to Queue__jki_lib_state_machine.vi"("State(s) in Front (\"\")"="Action: Import Calibration", "State(s) in (\"\")"=w124) -> ("States Out"=w125:string)  [unwired: 13 in]
          }
          event "Stop": Value Change {
            n54 = event-data() -> ()  [unwired: 1 in, 6 out]
            n55 = Release Queue(queue=w127, force destroy? (F)=TRUE) -> (error out=w129:errorcluster)  [unwired: 1 in, 2 out]
            n56 = call <vilib>:"Clear Errors.vi"("error in (no error)"=w129) -> ()  [unwired: 5 in, 2 out]
            n57 = call <vilib>:"Add State(s) to Queue__jki_lib_state_machine.vi"("State(s) in Front (\"\")"="Macro: Exit", "State(s) in (\"\")"=w134) -> ("States Out"=w133:string)  [unwired: 13 in]
          }
          event Panel Close? {
            n58 = event-data() -> ()  [unwired: 1 in, 1 out]
            n59 = property on="Stop" class="Bool (strict)"("Val(Sgnl)"=TRUE ("stop")) -> ()  [unwired: 2 in, 2 out]
            n60 = call <vilib>:"Add State(s) to Queue__jki_lib_state_machine.vi"("State(s) in (\"\")"=w140) -> ("States Out"=w139:string)  [unwired: 14 in]
            n61 = event-data("Discard?"=TRUE) -> ()  [unwired: 1 in, 1 out]
          }
        }
      }
      frame "---------- Core ----------" {
        # "Do not put any code in this frame.\n(it is a separator no-op)"
        n62 = call <vilib>:"Add State(s) to Queue__jki_lib_state_machine.vi"("State(s) in (\"\")"=w144) -> ("States Out"=w143:string)  [unwired: 14 in]
      }
      frame Default {
        w154 = 42 items=["No error", "Argument error", "Memory is full", "Out of zone", "End of file", "File already open", "Generic file I/O error", "File not found", "File permission error", "Disk is full", "Duplicate path", "Too many files open", "System feature not enabled", "Resource file not found", "Cannot add resource", "Resource not found", "Image not found", "Image memory error", "Pen does not exist", "Config type invalid", "Config token not found", "Config parse error", "Config memory error", "Bad external code format", "Bad external code offset", "External code not present", "Null window", "Destroy window error", "Null menu", "Print aborted", "Bad print record", "Print driver error", "Windows error during printing", "Memory error during printing", "Print dialog error", "Generic print error", "Invalid device refnum", "Device not found", "Device parameter error", "Device unit error", "Cannot open device", "Device call aborted", "Generic error", "Cancelled by user", "Object ID too low", "Object ID too high", "Object not in heap", "Unknown heap", "Unknown object (invalid DefProc)", "Unknown object (DefProc not in table)", "Message out of range", "Invalid (null) method", "Unknown message", "Manager call not supported", "Bad address", "Network operation in progress", "Network operation timed out", "Connection is busy", "Network attribute not supported", "Network error", "Address in use", "System out of memory", "Connection aborted", "Connection refused", "Not connected", "Already connected", "Connection closed", "Initialization error (interapplication manager)", "Bad occurrence", "Wait on unbound occurrence handler", "Occurrence queue overflow", "Datalog type conflict", "Unused", "Unrecognized type (interapplication manager)", "Memory corrupt", "Failed to make temporary DLL", "Old CIN version", "Drag socket not found", "Failed to load drop-object", "Failed to register OLE object", "Failed to release OLE object", "Format specifier type mismatch", "Unknown format specifier", "Too few format specifiers", "Too many format specifiers", "Scan failed", "Newer CIN version", "Error converting to variant", "Runtime menu error", "Password tampered", "Variant attribute not found", "Incompatible variant data type", "Event data is not available", "Event Store is not present", "Occurrence is not found", "Event Queue is not created", "Event info is not available", "Refnum passed is NULL", "Error retrieving Class GUID", "Error retrieving CoClass GUID", "Error retrieving TypeLib GUID.", "Bad built application magic bytes.", "Specific driver is different from the specific driver associated with the Logical Name.", "There is no session opened to the class driver.", "Max Error", "MAX - Error with config objects", "MAX - Error loading configuration", "MAX - Group not supported"]
        # "Current State"
        # "Do not delete, rename, or modify this frame.\n(this is used to capture unhandled states and typos)"
        # "Handle mistyped state name (developer tool)"
        n63 = Format Into String(format string="Software Exception: Unhandled State \"%s\"." ("message"), error in=w150, w145) -> (resulting string=w153:string, error out=w152:errorcluster)  [unwired: 1 in]
        n64 = call <vilib>:"Error Cluster From Error Code.vi"("show call chain? (False)"=TRUE, "error in (no error)"=w152, "error message (\"\")"=w153, "error code (0)"=w154) -> ("error out"=w151:errorcluster)  [unwired: 5 in]
        n65 = call <vilib>:"Add State(s) to Queue__jki_lib_state_machine.vi"("State(s) in (\"\")"=w149) -> ("States Out"=w148:string)  [unwired: 14 in]
      }
      frame "Initialize Core Data" {
        # "Do not delete, rename, or modify this frame.\n(this is used to determine panel behavior on exit)"
        # "originally closed?"
        # "exe?"
        # "If panel starts closed or is an EXE, then close it when we exit"
        n66 = property class="VI"() -> ("FP.State"=w158:T10)  [unwired: 2 in, 2 out]
        n67 = property class="App"() -> ("App.Kind"=w164:T11)  [unwired: 2 in, 2 out]
        n68 = control-ref of="Current VI Reference"() -> (w159:refnum<vi>)
        n69 = Equal?(x=w158, y=T10."Closed" ("Front Panel Window:State")) -> (x = y?=w156:bool)
        n70 = Equal?(x=w164, y=T11."Run Time System" ("Application:Kind")) -> (x = y?=w162:bool)
        n71 = Or(x=w156, y=w162) -> (x .or. y?=w160:bool)
        n72 = Bundle By Name(cluster=w161, "Core.Current VI Reference"=w159, "Core.Close Panel on Exit?"=w160) -> (w166:T13)
        n73 = call <vilib>:"Add State(s) to Queue__jki_lib_state_machine.vi"("State(s) in (\"\")"=w168) -> ("States Out"=w167:string)  [unwired: 14 in]
      }
      frame "Error Handler" {
        # "Unhandled Error -- Display it"
        # "Handle any errors here.\nYou can also output any states to clean-up after errors occur"
        # "Clear error"
        n74 = call <vilib>:"General Error Handler.vi"("error in (no error)"=w170) -> ()  [unwired: 10 in, 5 out]
        n75 = call <vilib>:"Add State(s) to Queue__jki_lib_state_machine.vi"("State(s) in Front (\"\")"="/* Post Error States", "State(s) in (\"\")"=w174) -> ("States Out"=w173:string)  [unwired: 13 in]
      }
      frame "Exit" {
        # "Do not put any code in this frame.\n(No errors that occur here will be handled.)"
        n76 = call <vilib>:"Add State(s) to Queue__jki_lib_state_machine.vi"("State(s) in (\"\")"=w179) -> ("States Out"=w178:string)  [unwired: 14 in]
      }
      frame "---------- Data ----------" {
        # "Do not put any code in this frame.\n(It is a separator no-op. You can make a copy of this frame to create a new Data frame)"
        n77 = call <vilib>:"Add State(s) to Queue__jki_lib_state_machine.vi"("State(s) in (\"\")"=w183) -> ("States Out"=w182:string)  [unwired: 14 in]
      }
      frame "Data: Initialize" {
        w184 = ""  # Diagnostic type
        w185 = T14 {"Hexapod zscan positions"=[], "Hexapod zscan diagnostic"=[], "Index"=0, "Best Zpos"=0.0}  # Hexapod zscan data
        w186 = cluster{"MaxCounts":dbl, "w0 Y":dbl} {"MaxCounts"=0.0, "w0 Y"=0.0}  # Beam diagnostic cutoffs
        w187 = cluster{"P1":string, "P2":string} {"P1"="", "P2"=""}  # Hexapod positions
        w188 = cluster{"T1":i32, "T2":i32} {"T1"=0, "T2"=0}  # Timer
        w189 = 0  # Alignment attempts
        w190 = 0  # Messages
        w193 = cluster{"X":dbl, "Y":dbl} {"X"=0.01, "Y"=0.02}  # Calibration Angle
        w194 = cluster{"X":dbl, "Y":dbl} {"X"=10.0, "Y"=10.0}  # Accuracy limit
        w195 = 8.0  # Calibration steps
        w196 = T15 {"Centroids.x"=[], "Centroids.y"=[]}  # Centroids
        w197 = cluster{"X":dbl, "Y":dbl} {"X"=0.0, "Y"=0.0}  # Scale Factor
        w198 = cluster{"X":dbl, "Y":dbl} {"X"=0.0, "Y"=0.0}  # Difference
        w199 = T16 {"Current VI Reference"=refnum, "Close Panel on Exit?"=FALSE}  # Core
        # "do not delete - used by framework"
        # "Data names and types of shift register data are defined by this bundle."
        # "Initialize the shift-register data, here.\n(data names are defined by what you wire into the bundle function)"
        n78 = call <vilib>:"Create.vi"("Settings"="Settings") -> ("NetworkConnection out"=w191:refnum<class "NetworkConnection.lvclass">)  [unwired: 9 in, 1 out]
        n79 = Bundle("Core"=w199, "Difference"=w198, "Scale Factor"=w197, "Centroids"=w196, "Calibration Angle"=w193, "Accuracy limit"=w194, "Calibration steps"=w195, "NetworkConnection out"=w191, "Messages"=w190, "Alignment attempts"=w189, "Timer"=w188, "Hexapod positions"=w187, "Beam diagnostic cutoffs"=w186, "Hexapod zscan data"=w185, "Diagnostic type"=w184) -> (w201:T13)  [unwired: 1 in]
        n80 = call <vilib>:"Add State(s) to Queue__jki_lib_state_machine.vi"("State(s) in (\"\")"=w203) -> ("States Out"=w202:string)  [unwired: 14 in]
      }
      frame "Data: Cleanup" {
        # "Cleanup any data and references, here.\n(this is called automatically, by the Macro: Exit)"
        n81 = Unbundle By Name(w207) -> ("Core.Current VI Reference"=w209:refnum<vi>)
        n82 = Close Reference(reference=w209, error in (no error)=w208) -> (error out=w205:errorcluster)
        n83 = Unbundle By Name(w207) -> ("NetworkConnection out"=w206:refnum<class "NetworkConnection.lvclass">)
        n84 = call <vilib>:"Destroy.vi"("error in (no error)"=w205, "NetworkConnection in"=w206) -> ("error out"=w204:errorcluster)  [unwired: 8 in, 1 out]
        n85 = call <vilib>:"Add State(s) to Queue__jki_lib_state_machine.vi"("State(s) in (\"\")"=w211) -> ("States Out"=w210:string)  [unwired: 14 in]
      }
      frame "---------- UI ----------" {
        # "Do not put any code in this frame.\n(It is a separator no-op. You can make a copy of this frame to create a new UI frame)"
        n86 = call <vilib>:"Add State(s) to Queue__jki_lib_state_machine.vi"("State(s) in (\"\")"=w215) -> ("States Out"=w214:string)  [unwired: 14 in]
      }
      frame "UI: Initialize" {
        # "Initialize the User Interface, here.\n(this is called automatically, by the Macro: Init)"
        n87 = call <vilib>:"Add State(s) to Queue__jki_lib_state_machine.vi"("State(s) in (\"\")"=w219) -> ("States Out"=w218:string)  [unwired: 14 in]
      }
      frame "UI: Cursor Set" {
        # "Argument"
        # "Set and Unset Cursor Busy.\n(Usage: \"UI: Cursor Set >> Busy|Idle\")"
        n88 = case shown="\"Idle\", Default" w220 {
          tunnel: w222 -> [w227 w229]
          tunnel: [w226 w228] -> w221
          frame "Idle", Default {
            n89 = call <vilib>:"Unset Busy.vi"("error in (no error)"=w227) -> ("error out"=w226:errorcluster)  [unwired: 10 in]
          }
          frame "Busy" {
            n90 = call <vilib>:"Set Busy.vi"("error in (no error)"=w229) -> ("error out"=w228:errorcluster)  [unwired: 9 in, 1 out]
          }
        }
        n91 = call <vilib>:"Add State(s) to Queue__jki_lib_state_machine.vi"("State(s) in (\"\")"=w225) -> ("States Out"=w224:string)  [unwired: 14 in]
      }
      frame "UI: Front Panel State" {
        # "Argument"
        # "Set Front Panel Open or Closed\n(Usage: \"UI: Front Panel State >> Open|Close\")"
        n92 = Unbundle By Name(w232) -> ("Core.Current VI Reference"=w231:refnum<vi>)
        n93 = case shown="\"Close\", \"Closed\"" w230 {
          tunnel: w234 -> [w242 w257 w268 w281 w294]
          tunnel: [w244 w258 w270 w283 w296] -> w233
          tunnel: w231 -> [w243 w255 w269 w282 w295]
          frame "Open", "Standard", Default {
            w237 = T10."Standard" ("State")
            n94 = property class="VI"(reference=w243, error in=w242) -> (reference out=w240:refnum<vi>, error out=w241:errorcluster, "FP.State"=w239:T10)
            n95 = Not Equal?(x=w239, y=w237) -> (x != y?=w238:bool)
            n96 = case shown="True" w238 {
              tunnel: [w248 w250] -> w244
              tunnel: w241 -> [w247 w250]
              tunnel: w240 -> [w246 _]
              tunnel: w237 -> [w245 _]
              frame True {
                n97 = invoke class="VI" method="FP.Open"(reference=w246, error in=w247, "Activate"=TRUE, "State"=w245) -> (error out=w248:errorcluster)  [unwired: 1 in, 4 out]
              }
              frame False {
              }
            }
          }
          frame "Close", "Closed" {
            n98 = property class="VI"(reference=w255, error in=w257) -> (reference out=w254:refnum<vi>, error out=w256:errorcluster, "FP.State"=w252:T10)
            n99 = Not Equal?(x=w252, y=T10."Closed" ("Front Panel Window:State")) -> (x != y?=w251:bool)
            n100 = case shown="False" w251 {
              tunnel: [w259 w262] -> w258
              tunnel: w256 -> [w259 w261]
              tunnel: w254 -> [_ w260]
              frame False {
              }
              frame True {
                n101 = invoke class="VI" method="FP.Close"(reference=w260, error in=w261) -> (error out=w262:errorcluster)  [unwired: 1 in, 2 out]
              }
            }
          }
          frame "Hidden", "Hide" {
            w263 = T10."Hidden" ("State")
            n102 = property class="VI"(reference=w269, error in=w268) -> (reference out=w266:refnum<vi>, error out=w267:errorcluster, "FP.State"=w265:T10)
            n103 = Not Equal?(x=w265, y=w263) -> (x != y?=w264:bool)
            n104 = case shown="True" w264 {
              tunnel: [w274 w275] -> w270
              tunnel: w267 -> [w273 w275]
              tunnel: w266 -> [w272 _]
              tunnel: w263 -> [w271 _]
              frame True {
                n105 = invoke class="VI" method="FP.Open"(reference=w272, error in=w273, "State"=w271) -> (error out=w274:errorcluster)  [unwired: 2 in, 4 out]
              }
              frame False {
              }
            }
          }
          frame "Minimize", "Minimized" {
            w276 = T10."Minimized" ("State")
            n106 = property class="VI"(reference=w282, error in=w281) -> (reference out=w279:refnum<vi>, error out=w280:errorcluster, "FP.State"=w278:T10)
            n107 = Not Equal?(x=w278, y=w276) -> (x != y?=w277:bool)
            n108 = case shown="True" w277 {
              tunnel: [w287 w288] -> w283
              tunnel: w280 -> [w286 w288]
              tunnel: w279 -> [w285 _]
              tunnel: w276 -> [w284 _]
              frame True {
                n109 = invoke class="VI" method="FP.Open"(reference=w285, error in=w286, "State"=w284) -> (error out=w287:errorcluster)  [unwired: 2 in, 4 out]
              }
              frame False {
              }
            }
          }
          frame "Maximize", "Maximized" {
            w289 = T10."Maximized" ("State")
            n110 = property class="VI"(reference=w295, error in=w294) -> (reference out=w292:refnum<vi>, error out=w293:errorcluster, "FP.State"=w291:T10)
            n111 = Not Equal?(x=w291, y=w289) -> (x != y?=w290:bool)
            n112 = case shown="True" w290 {
              tunnel: [w300 w301] -> w296
              tunnel: w293 -> [w299 w301]
              tunnel: w292 -> [w298 _]
              tunnel: w289 -> [w297 _]
              frame True {
                n113 = invoke class="VI" method="FP.Open"(reference=w298, error in=w299, "State"=w297) -> (error out=w300:errorcluster)  [unwired: 2 in, 4 out]
              }
              frame False {
              }
            }
          }
        }
        n114 = call <vilib>:"Add State(s) to Queue__jki_lib_state_machine.vi"("State(s) in (\"\")"=w236) -> ("States Out"=w235:string)  [unwired: 14 in]
      }
      frame "---------- Macro ----------" {
        # "Do not put any code in this frame.\n(It is a separator no-op. You can make a copy of this frame to create a new Macro frame)"
        n115 = call <vilib>:"Add State(s) to Queue__jki_lib_state_machine.vi"("State(s) in (\"\")"=w305) -> ("States Out"=w304:string)  [unwired: 14 in]
      }
      frame "Macro: Initialize" {
        # "Initialization Macro\n(This is called once, when the VI starts)"
        n116 = call <vilib>:"Add State(s) to Queue__jki_lib_state_machine.vi"("State(s) in Front (\"\")"="Data: Initialize\nInitialize Core Data\nUI: Initialize\nUI: Front Panel State >> Open\nAction: Import Calibration", "State(s) in (\"\")"=w310) -> ("States Out"=w309:string)  [unwired: 13 in]
      }
      frame "Macro: Calibrate" {
        w312 = dbl[] []
        # "Create the state list for calibration"
        # "Empty the array"
        n117 = Unbundle By Name(w313) -> ("Calibration steps"=w314:dbl)
        n118 = call <vilib>:"Add State(s) to Queue__jki_lib_state_machine.vi"("State(s) in Front (\"\")"="Action: Get Centroid>> Calibrate", "State(s) in (\"\")"=w320) -> ("States Out"=w319:string)  [unwired: 13 in]
        n119 = Subtract(x=w314, y=1.0) -> (x-y=w317:dbl)
        n120 = for {
          N: w317 -> [_]
          shift-right: [w324] -> w315
          shift-left: w319 -> [w326]
          n121 = call <vilib>:"Add State(s) to Queue__jki_lib_state_machine.vi"("State(s) in (\"\")"=w326, "State(s) at Back (\"\")"="Action: Move>> Calibrate\nAction: Get Centroid>> Calibrate") -> ("States Out"=w324:string)  [unwired: 13 in]
        }
        n122 = call <vilib>:"Add State(s) to Queue__jki_lib_state_machine.vi"("State(s) in (\"\")"=w315, "State(s) at Back (\"\")"="Action: Calibrate" ("State(s) in Front (\"\")")) -> ("States Out"=w323:string)  [unwired: 13 in]
        n123 = Bundle By Name(cluster=w313, "Centroids.Centroids.x"=w312, "Centroids.Centroids.y"=w312) -> (w311:T13)
      }
      frame "Macro: Hexapod Zpos Scan" {
        n124 = In Range and Coerce(upper limit="central z upper limit", x="Central position of z scan", lower limit="central z lower limit") -> (coerced(x)=w327:dbl)  [unwired: 1 out]
        n125 = case shown="\"w0 Y\"" "Diagnostic type" {
          tunnel: ["maxcounts" "w0y"] -> w336
          frame "Max counts", Default {
          }
          frame "w0 Y" {
          }
        }
        n126 = Divide(x="zpos scan range", y=2) -> (x/y=w345:dbl)
        n127 = Divide(x="zpos scan range", y="zpos scan increment") -> (x/y=w350:dbl)
        n128 = Subtract(x=w327, y=w345) -> (x-y=w344:dbl)
        n129 = Increment(x=w350) -> (x+1=w341:dbl)
        n130 = for {
          N: w341 -> [_]
          tunnel: [w363] -> w333 mode=indexing
          i -> [w363]
        }
        n131 = Array Size(array=w333) -> (size(s)=w332:i32)
        n132 = Multiply(x=w333, y="zpos scan increment") -> (x*y=w348:dbl[])
        n133 = Add(x=w344, y=w348) -> (x+y=w331:dbl[])
        n134 = for {
          N: w332 -> [_]
          shift-right: [w362] -> w335
          shift-left: w339 -> [w361]
          tunnel: w331 -> [w359] mode=indexing
          n135 = Number To Fractional String(number=w359) -> (F-format string=w357:string)  [unwired: 3 in]
          n136 = call <vilib>:"Build State String with Arguments__JKI_lib_State_Machine.vi"("Arguments (\"\")"=w357, "State"="Action: Move>> Zpos Scan") -> ("State with Arguments"=w356:string)  [unwired: 4 in]
          n137 = call <vilib>:"Add State(s) to Queue__jki_lib_state_machine.vi"("State(s) in Front (\"\")"=w356, "State(s) in (\"\")"="Action: Get Beam Diagnostic>>Zpos Scan", "State(s) at Back (\"\")"=w361) -> ("States Out"=w362:string)  [unwired: 12 in]
        }
        n138 = disable-structure shown="Disabled" {
          frame Disabled {
            n139 = local read "Newmark for vertical"() -> (w353:bool)
            n140 = case shown="True" w353 {
              frame False {
              }
              frame True {
                n141 = local read "zpos::2"() -> ()  [unwired: 1 out]
              }
            }
          }
          frame Enabled {
          }
        }
        n142 = Bundle By Name(cluster=w343, "Hexapod zscan data.Hexapod zscan positions"=w331, "Hexapod zscan data.Index"=0, "Hexapod zscan data.Hexapod zscan diagnostic"=dbl[] [], "Diagnostic type"=w336) -> (w342:T13)
        n143 = call <vilib>:"Add State(s) to Queue__jki_lib_state_machine.vi"("State(s) in Front (\"\")"=w335, "State(s) in (\"\")"="Action: Find Best Zpos") -> ("States Out"=w352:string)  [unwired: 13 in]
      }
      frame "Macro: Alignment" {
        n144 = call <userlib>:"Wait (ms)__ogtk.vi"("milliseconds to wait"=u32 300) -> ("error out"=w366:errorcluster)  [unwired: 9 in, 1 out]
        n145 = flat-sequence {
          tunnel: [w378] -> w367
          tunnel: w366 -> [_]
          tunnel: [w375] -> w364
          frame #0 {
            n146 = local read "Disable pointing correction"() -> (w378:bool)
            n147 = local read "MaxCounts::1"() -> (w377:dbl)
            n148 = Greater?(x=w377, y="Min counts for align") -> (0:w375:bool)
            "Max counts ok align" <- w375
          }
        }
        n149 = case shown="False" w367 {
          tunnel: [w380 w382] -> w371
          tunnel: w364 -> [w379 w383]
          frame False {
            # "pointing not disabled"
            n150 = case shown="True" w379 {
              tunnel: [_ "Update: Alignment Constants\nAction: Get Centroid>> Align"] -> w380
              frame False {
              }
              frame True {
                # "Create initial state list for alignment"
                # "counts high enough to align"
              }
            }
          }
          frame True {
            # "pointning disabled"
            n151 = case shown="True" w383 {
              tunnel: [_ " Action: Send Response "] -> w382
              frame False {
              }
              frame True {
                # "counts high enough"
              }
            }
          }
        }
        n152 = Tick Count (ms)() -> (millisecond timer value=w370:u32)
        n153 = Bundle By Name(cluster=w368, "Timer.T1"=w370) -> (w369:T13)
        n154 = call <vilib>:"Add State(s) to Queue__jki_lib_state_machine.vi"("State(s) in Front (\"\")"=w371, "State(s) in (\"\")"=w372) -> ("States Out"=w374:string)  [unwired: 13 in]
      }
      frame "Macro: Exit" {
        # "Exit Macro\n(This is called once, when the VI exits)"
        n155 = disable-structure shown="Enabled" {
          disable-tunnel: w391 -> [w396 _]
          disable-tunnel: [w395 FALSE ("Close Panel on Exit?")] -> w386
          frame Disabled {
            n156 = Unbundle By Name(w396) -> ("Core.Close Panel on Exit?"=w395:bool)
          }
          frame Enabled {
          }
        }
        n157 = Select(t="UI: Front Panel State >> Close", s=w386, f="") -> (s? t:f=w389:string)
        n158 = call <vilib>:"Add State(s) to Queue__jki_lib_state_machine.vi"("State(s) in (\"\")"=w389, "State(s) at Back (\"\")"="Data: Cleanup\nExit") -> ("States Out"=w387:string)  [unwired: 13 in]
        n159 = call <vilib>:"Add State(s) to Queue__jki_lib_state_machine.vi"("State(s) in Front (\"\")"=w387, "State(s) in (\"\")"=w394) -> ("States Out"=w393:string)  [unwired: 13 in]
      }
      frame "---------- Update ----------" {
        # "Do not put any code in this frame.\n(It is a separator no-op. You can make a copy of this frame to create a new Macro frame)"
        n160 = call <vilib>:"Add State(s) to Queue__jki_lib_state_machine.vi"("State(s) in (\"\")"=w401) -> ("States Out"=w400:string)  [unwired: 14 in]
      }
      frame "Update: Calibration Constants" {
        n161 = Bundle By Name(cluster=w405, "Calibration steps"="Calibration steps", "Calibration Angle"="Calibration Angle", "Alignment attempts"=0) -> (w404:T13)
        n162 = call <vilib>:"Add State(s) to Queue__jki_lib_state_machine.vi"("State(s) in (\"\")"=w407) -> ("States Out"=w409:string)  [unwired: 14 in]
      }
      frame "Update: Alignment Constants" {
        n163 = Bundle By Name(cluster=w414, "Accuracy limit"="Accuracy limit", "Alignment attempts"=0) -> (w413:T13)
        n164 = call <vilib>:"Add State(s) to Queue__jki_lib_state_machine.vi"("State(s) in (\"\")"=w415) -> ("States Out"=w416:string)  [unwired: 14 in]
      }
      frame "---------- Action ----------" {
        # "Do not put any code in this frame.\n(It is a separator no-op. You can make a copy of this frame to create a new Macro frame)"
        n165 = call <vilib>:"Add State(s) to Queue__jki_lib_state_machine.vi"("State(s) in (\"\")"=w420) -> ("States Out"=w419:string)  [unwired: 14 in]
      }
      frame "Action: Get Centroid" {
        n166 = call <userlib>:"Wait (ms)__ogtk.vi"("error in (no error)"=w423, "milliseconds to wait"=u32 600) -> ("error out"=w422:errorcluster)  [unwired: 8 in, 1 out]
        n167 = flat-sequence {
          tunnel: ["Target.X::1"] -> w430
          tunnel: ["Target.Y::1"] -> w429
          tunnel: ["centroidx::1"] -> w428
          tunnel: ["centroidy::1"] -> w427
          tunnel: w422 -> [_]
          frame #0 {
          }
        }
        n168 = case shown="\"Align\", Default" w424 {
          tunnel: w425 -> [w442 w467]
          tunnel: w427 -> [w444 w454]
          tunnel: w428 -> [w443 w453]
          tunnel: [w441 w463] -> w432
          tunnel: w430 -> [_ w466]
          tunnel: w429 -> [_ w465]
          tunnel: ["" w464] -> w431
          tunnel: w423 -> [w439 w452]
          tunnel: [w439 w452] -> w426
          frame "Calibrate" {
            # "Reads centroid position and adds them to array for calibration calculation"
            n169 = Unbundle By Name(w442) -> ("Centroids.Centroids.x"=w445:dbl[], "Centroids.Centroids.y"=w446:dbl[])
            n170 = Build Array (concatenate)(w445, w443) -> (w447:dbl[])
            n171 = Build Array (concatenate)(w446, w444) -> (w448:dbl[])
            n172 = Bundle By Name(cluster=w442, "Centroids.Centroids.x"=w447, "Centroids.Centroids.y"=w448) -> (w441:T13)
          }
          frame "Align", Default {
            # "After movement, check if difference between centroid and target is within tolerance. If it is within tolerance, end alignment. If it isn't within tolerance, move hexapod again."
            n173 = Unbundle By Name(w467) -> ("Accuracy limit.X"=w462:dbl, "Accuracy limit.Y"=w460:dbl)
            n174 = Subtract(x=w466, y=w453) -> (x-y=w469:dbl)
            n175 = Subtract(x=w465, y=w454) -> (x-y=w468:dbl)
            n176 = Bundle By Name(cluster=w467, "Difference.X"=w469, "Difference.Y"=w468) -> (w463:T13)
            n177 = Absolute Value(x=w469) -> (abs(x)=w461:dbl)
            n178 = Absolute Value(x=w468) -> (abs(x)=w459:dbl)
            n179 = local read "Disable pointing correction"() -> (w451:bool)
            n180 = Greater?(x=w462, y=w461) -> (0:w455:bool)
            n181 = Greater?(x=w460, y=w459) -> (0:w456:bool)
            n182 = And(x=w455, y=w456) -> (x .and. y?=w450:bool)
            n183 = Or(x=w451, y=w450) -> (x .or. y?=w449:bool)
            n184 = Select(t=" Action: Send Response ", s=w449, f="Action: Move>> Align\nAction: Get Centroid>> Align") -> (s? t:f=w464:string)
            n185 = case shown="True" w449 {
              tunnel: w454 -> [_ w473]
              tunnel: w453 -> [_ w471]
              frame False {
              }
              frame True {
                n186 = Bundle("centroidx::1"=w471, "centroidy::1"=w473) -> (→"Waveform Chart":cluster{"centroidx::1":dbl, "centroidy::1":dbl})  [unwired: 1 in]
                n187 = local write "tab"(T9."Controls" ("tab")) -> ()
              }
            }
          }
        }
        n188 = call <vilib>:"Add State(s) to Queue__jki_lib_state_machine.vi"("State(s) in Front (\"\")"=w431, "State(s) in (\"\")"=w434) -> ("States Out"=w433:string)  [unwired: 13 in]
      }
      frame "Action: Move" {
        # "send movement command to hexapod\nand wait for slow response"
        n189 = call "get arguments of jki state.vi"("jki arguments"=w476, "spaces around >>"=TRUE) -> ("Arg 1"=w478:string)  [unwired: 2 out]
        n190 = case shown="\"Align\", Default" w478 {
          tunnel: w502 -> [w563 w593 w617 w627]
          tunnel: "xpos::2" -> [w574 w604 w625 w634]
          tunnel: [w574 w604 w625 w634] -> w493
          tunnel: "ypos::2" -> [w573 w603 w624 w633]
          tunnel: [w573 w603 w624 w633] -> w491
          tunnel: "zpos::2" -> [w565 w602 _ _]
          tunnel: [w565 w602 w616 w629] -> w489
          tunnel: "uangle::2" -> [w566 w599 w623 w632]
          tunnel: [w566 w599 w623 w632] -> w487
          tunnel: "wangle::2" -> [w571 w575 w621 w630]
          tunnel: [w570 w576 w621 w630] -> w485
          tunnel: "vangle::2" -> [w568 w580 w622 w631]
          tunnel: [w567 w579 w622 w631] -> w483
          tunnel: w477 -> [w564 w595 w618 w628]
          tunnel: [w564 w592 w618 w628] -> w482
          tunnel: [w563 w591 w617 w627] -> w481
          tunnel: [FALSE ("Hex for vertical") FALSE ("Hex for vertical") TRUE ("Hex for vertical") TRUE ("Hex for vertical")] -> w474
          frame "Calibrate" {
            # "Calibration movement"
            n191 = Unbundle By Name(w563) -> ("Calibration Angle.Y"=w569:dbl, "Calibration Angle.X"=w572:dbl)
            n192 = Add(x=w568, y=w569) -> (x+y=w567:dbl)
            n193 = Add(x=w572, y=w571) -> (x+y=w570:dbl)
          }
          frame "Align", Default {
            # "Correction movement, scaled by a factor"
            n194 = Unbundle By Name(w593) -> ("Alignment attempts"=w596:i32)
            n195 = Unbundle By Name(w593) -> ("Difference.Y"=w611:dbl, "Scale Factor.Y"=w610:dbl, "Difference.X"=w609:dbl, "Scale Factor.X"=w608:dbl)
            n196 = Multiply(x=w609, y=w608) -> (x*y=w606:dbl)
            n197 = Multiply(x=w611, y=w610) -> (x*y=w607:dbl)
            n198 = Increment(x=w596) -> (x+1=w598:i32)
            "Alignment attempts" <- w598
            n199 = Multiply(x="Buffer", y=w606) -> (x*y=w601:dbl)
            n200 = Multiply(x=w607, y="Buffer") -> (x*y=w600:dbl)
            n201 = Add(x=w601, y=w575) -> (x+y=w587:dbl)
            n202 = Add(x=w600, y=w580) -> (x+y=w588:dbl)
            n203 = Greater?(x=w598, y=10) -> (0:w597:bool)
            n204 = case shown="True" w597 {
              tunnel: [w612 ""] -> w592
              tunnel: w595 -> [w612 _]
              frame False {
              }
              frame True {
                (unwired) " Action: Send Response "
                # "align failed. notify tAPE?"
              }
            }
            n205 = Bundle By Name(cluster=w593, "Alignment attempts"=w598) -> (w591:T13)
            n206 = local write "tab"(T9."Data" ("tab")) -> ()
            n207 = In Range and Coerce(upper limit="vangle upper limit", x=w588, lower limit="vangle lower limit") -> (coerced(x)=w581:dbl, In Range?=w582:bool)
            "move In Range V" <- w582
            n208 = In Range and Coerce(upper limit="wangle upper limit", x=w587, lower limit="wangle lower limit") -> (coerced(x)=w577:dbl, In Range?=w578:bool)
            "move In Range W" <- w578
            n209 = Select(t=w581, s=w582, f=w580) -> (s? t:f=w579:dbl)
            n210 = Select(t=w577, s=w578, f=w575) -> (s? t:f=w576:dbl)
          }
          frame "Zpos Scan" {
            n211 = Unbundle By Name(w617) -> ("Hexapod zscan data.Index"=w620:i32, "Hexapod zscan data.Hexapod zscan positions"=w619:dbl[])
            n212 = Index Array(array=w619, index=w620) -> (element=w616:dbl)
            n213 = local write "tab"(T9."Z scan" ("tab")) -> ()
          }
          frame "Best Zpos" {
            n214 = Unbundle By Name(w627) -> ("Hexapod zscan data.Best Zpos"=w629:dbl)
          }
        }
        n215 = call <userlib>:"Tick Count (ms)__ogtk.vi"("error in (no error)"=w501) -> ("error out"=w497:errorcluster, "millisecond timer value"=w499:u32)  [unwired: 9 in]
        n216 = disable-structure "Diagram Disable Structure" shown="Enabled" {
          disable-tunnel: w493 -> [w519 _]
          disable-tunnel: w491 -> [w518 _]
          disable-tunnel: w489 -> [w517 _]
          disable-tunnel: w487 -> [w516 _]
          disable-tunnel: w483 -> [w515 w557]
          disable-tunnel: w485 -> [w514 w558]
          disable-tunnel: "GUIdevice 2" -> [w509 w554]
          disable-tunnel: w497 -> [w513 w561]
          disable-tunnel: [w511 w559] -> w496
          disable-tunnel: "Newmark for vertical" -> [w505 _]
          disable-tunnel: w474 -> [w506 _]
          frame Enabled {
            # "Full xyzuvw command structure"
            n217 = And(x=w505, y=w506) -> (x .and. y?=w504:bool)
            n218 = case shown="True" w504 {
              tunnel: w519 -> [w539 _]
              tunnel: w518 -> [w538 _]
              tunnel: w517 -> [w537 w544]
              tunnel: w516 -> [w536 _]
              tunnel: w515 -> [w535 _]
              tunnel: w514 -> [w534 _]
              tunnel: [w528 w546] -> w512
              tunnel: w509 -> [w527 _]
              tunnel: [w527 "GUIdevice 3"] -> w508
              tunnel: [TRUE TRUE] -> w507
              frame False {
                # "create command"
                # "turn into proper formatting"
                # "convert to string"
                # "create hexapod state array"
                n219 = Build Array(w539, w538, w537, w536, w535, w534) -> (w533:dbl[])
                n220 = Number To Fractional String(number=w533) -> (F-format string=w532:string[])  [unwired: 3 in]
                n221 = call <userlib>:"1D Array to String__ogtk.vi"("delimiter (Tab)"="," ("string"), "Array of Strings"=w532) -> ("delimited string"=w529:string)  [unwired: 9 in]
                n222 = Concatenate Strings("setxyzuvw>>" ("command in"), w529) -> (w528:string)
              }
              frame True {
                # "race!!!"
                n223 = Subtract(x=w544, y="position::3") -> (x-y=w543:dbl)
                n224 = Number To Fractional String(number=w544) -> (F-format string=w547:string)  [unwired: 3 in]
                n225 = Absolute Value(x=w543) -> (abs(x)=w542:dbl)
                n226 = Concatenate Strings("setposition>>" ("command in"), w547) -> (w546:string)
                n227 = Greater?(x=w542, y=0.05) -> ()  [unwired: 1 out]
              }
            }
            n228 = case shown="True" w507 {
              tunnel: w513 -> [w520 w525]
              tunnel: w512 -> [_ w524]
              tunnel: [w520 w523] -> w511
              tunnel: [_ w522] -> w510
              tunnel: w508 -> [_ w521]
              frame False {
              }
              frame True {
                n229 = call "send udp and wait for slow response.vi"("error in"=w525, "command in"=w524, "Device"=w521) -> ("error out"=w523:errorcluster, "slow response"=w522:string)  [unwired: 4 in, 3 out]
              }
            }
            "slow response" <- w510
          }
          frame Disabled {
            # "separate w and v angle commands"
            n230 = Number To Fractional String(number=w558) -> (F-format string=w555:string)  [unwired: 3 in]
            n231 = Number To Fractional String(number=w557) -> (F-format string=w552:string)  [unwired: 3 in]
            n232 = Concatenate Strings("setwangle >>", w555) -> (w553:string)
            n233 = Concatenate Strings("setvangle>>", w552) -> (w550:string)
            n234 = call "send udp and wait for slow response.vi"("error in"=w561, "command in"=w553, "Device"=w554) -> ("error out"=w560:errorcluster)  [unwired: 4 in, 4 out]
            n235 = call "send udp and wait for slow response.vi"("error in"=w560, "command in"=w550, "Device"=w554) -> ("error out"=w559:errorcluster)  [unwired: 4 in, 4 out]
          }
        }
        n236 = call <userlib>:"Tick Count (ms)__ogtk.vi"("error in (no error)"=w496) -> ("error out"=w495:errorcluster, "millisecond timer value"=w500:u32)  [unwired: 9 in]
        n237 = Subtract(x=w500, y=w499) -> (x-y=→"Waveform Chart 2" →"Movement time":u32)
        n238 = call <vilib>:"Add State(s) to Queue__jki_lib_state_machine.vi"("State(s) in (\"\")"=w482) -> ("States Out"=w503:string)  [unwired: 14 in]
      }
      frame "Action: Calibrate" {
        # "Same as below but for x data"
        # "linear regression fit of data"
        # "cluster of best fit data"
        # "cluster of actual data"
        # "Create array of calibration steps"
        n239 = Unbundle By Name(w655) -> ("Calibration steps"=w648:dbl, "Calibration Angle.X"=w654:dbl, "Centroids.Centroids.x"=w638:dbl[], "Calibration Angle.Y"=w637:dbl, "Centroids.Centroids.y"=w647:dbl[])
        n240 = for {
          N: w648 -> [_]
          tunnel: [w660] -> w653 mode=indexing
          i -> [w660]
        }
        n241 = Multiply(x=w653, y=w637) -> (x*y=w651:dbl[])
        n242 = Multiply(x=w654, y=w653) -> (x*y=w652:dbl[])
        n243 = Bundle("Centroids.x"=w638, w652) -> (w643:cluster{"Centroids.x":dbl[], dbl[]})  [unwired: 1 in]
        n244 = call <vilib>:"Linear Fit.vi"("Y"=w652, "X"=w638) -> ("Best Linear Fit"=w635:dbl[], "slope"=w650:dbl, "residue"=→"X error":dbl)  [unwired: 9 in, 2 out]
        "X slope" <- w650
        n245 = Bundle("Centroids.y"=w647, w651) -> (w645:cluster{"Centroids.y":dbl[], dbl[]})  [unwired: 1 in]
        n246 = call <vilib>:"Linear Fit.vi"("Y"=w651, "X"=w647) -> ("Best Linear Fit"=w636:dbl[], "slope"=w649:dbl, "residue"=→"Y error":dbl)  [unwired: 9 in, 2 out]
        "Y slope" <- w649
        n247 = Bundle("Centroids.x"=w638, "Best Linear Fit"=w635) -> (w642:T17)  [unwired: 1 in]
        n248 = Bundle("Centroids.y"=w647, "Best Linear Fit"=w636) -> (w646:T18)  [unwired: 1 in]
        n249 = Build Array(w643, w642) -> (→"X Graph":T2)
        n250 = Build Array(w645, w646) -> (→"Y Graph":T3)
        n251 = Bundle By Name(cluster=w655, "Scale Factor.X"=w650, "Scale Factor.Y"=w649) -> (w656:T13)
        n252 = call <vilib>:"Add State(s) to Queue__jki_lib_state_machine.vi"("State(s) in (\"\")"=w659) -> ("States Out"=w658:string)  [unwired: 14 in]
      }
      frame "Action: Export Calibration" {
        n253 = Unbundle By Name(w665) -> ("Scale Factor"=w664:cluster{"X":dbl, "Y":dbl})
        n254 = call <userlib>:"MGI Write Anything.vi"("Error In"=w662, "Section Name (Name of \"Anything\")"="Calibration", "Anything"=w664) -> ("Error Out"=w661:errorcluster)  [unwired: 6 in, 2 out]
        n255 = call <vilib>:"Add State(s) to Queue__jki_lib_state_machine.vi"("State(s) in (\"\")"=w667) -> ("States Out"=w666:string)  [unwired: 14 in]
      }
      frame "Action: Import Calibration" {
        n256 = Unbundle By Name(w673) -> ("Scale Factor"=w672:cluster{"X":dbl, "Y":dbl})
        n257 = call <userlib>:"MGI Read Anything.vi"("Type of Anything"=w672, "Error In"=w669, "Section Name (Name of \"Type of Anything\")"="Calibration") -> ("Error Out"=w675:errorcluster, "Anything"=w674:variant)  [unwired: 5 in, 2 out]
        n258 = Variant To Data(error in=w675, type=w672, Variant=w674) -> (data=w671:cluster{"X":dbl, "Y":dbl}, error out=w668:errorcluster)
        n259 = Bundle By Name(cluster=w673, "Scale Factor"=w671) -> (w676:T13)
        n260 = call <vilib>:"Add State(s) to Queue__jki_lib_state_machine.vi"("State(s) in (\"\")"=w678) -> ("States Out"=w677:string)  [unwired: 14 in]
      }
      frame "Action: Get Beam Diagnostic" {
        n261 = Unbundle By Name(w684) -> ("Diagnostic type"=w683:string)
        n262 = call <userlib>:"Wait (ms)__ogtk.vi"("milliseconds to wait"=u32 250) -> ("error out"=w682:errorcluster)  [unwired: 9 in, 1 out]
        n263 = case shown="\"maxcounts\", Default" w683 {
          tunnel: ["MaxCounts::1" "2ndmomW0y::1"] -> w689
          tunnel: w682 -> [_ _]
          frame "maxcounts", Default {
          }
          frame "w0y" {
          }
        }
        n264 = case shown="\"Check Quality\", Default" w690 {
          tunnel: w684 -> [w703 w737]
          tunnel: w689 -> [w697 w727]
          tunnel: [w699 ""] -> w688
          tunnel: [w703 w731] -> w687
          tunnel: w686 -> [w702 w735]
          tunnel: [w702 w735] -> w685
          tunnel: w680 -> [w694 w730]
          tunnel: [w694 w728] -> w679
          frame "Check Quality", Default {
            # "#todo these should be separated so can check counts after. i.e. in macro alignment"
            n265 = Not(x="Disable pointing correction") -> (.not. x?=w695:bool)
            n266 = case shown="False" "always z scan" {
              tunnel: w697 -> [w707 _]
              tunnel: [w710 "Macro: Hexapod Zpos Scan"] -> w701
              tunnel: w695 -> [w709 _]
              frame False {
                n267 = In Range and Coerce(upper limit="Dont z scan if above this counts", x=w707, lower limit="Min counts for z scan") -> (In Range?=w705:bool)  [unwired: 1 out]
                "ZCounts In Range?" <- w705
                n268 = case shown="True" w705 {
                  tunnel: [w711 w717] -> w710
                  tunnel: w709 -> [w712 w715]
                  tunnel: "Disable Zpos Scan" -> [_ w716]
                  frame False {
                    n269 = case shown="True" w712 {
                      tunnel: ["" "Macro: Alignment"] -> w711
                      frame False {
                      }
                      frame True {
                      }
                    }
                  }
                  frame True {
                    n270 = case shown="True" w716 {
                      tunnel: ["Macro: Hexapod Zpos Scan" w720] -> w717
                      tunnel: w715 -> [_ w719]
                      frame False {
                      }
                      frame True {
                        n271 = case shown="True" w719 {
                          tunnel: [_ "Macro: Alignment"] -> w720
                          frame False {
                          }
                          frame True {
                          }
                        }
                      }
                    }
                  }
                }
              }
              frame True {
              }
            }
            n272 = call <vilib>:"Add State(s) to Queue__jki_lib_state_machine.vi"("State(s) in Front (\"\")"=w701) -> ("States Out"=w699:string)  [unwired: 14 in]
            "msg" <- w699
            n273 = local write "tab"(T1."message" ("tab")) -> ()
          }
          frame "Zpos Scan" {
            n274 = Unbundle By Name(w737) -> ("Hexapod zscan data.Hexapod zscan diagnostic"=w741:dbl[], "Hexapod zscan data.Index"=w739:i32)
            n275 = Greater Or Equal?(x=w727, y=4040.0) -> (x >= y?=w725:bool)
            n276 = Build Array (concatenate)(w741, w727) -> (w740:dbl[])
            n277 = Increment(x=w739) -> (x+1=w738:i32)
            n278 = Bundle By Name(cluster=w737, "Hexapod zscan data.Hexapod zscan diagnostic"=w740, "Hexapod zscan data.Index"=w738) -> (w731:T13)
            n279 = Unbundle By Name(w731) -> ("Hexapod zscan data.Hexapod zscan positions"=w733:dbl[], "Hexapod zscan data.Hexapod zscan diagnostic"=w732:dbl[])
            n280 = Bundle("Hexapod zscan positions"=w733, "Hexapod zscan diagnostic"=w732) -> (w734:T6)  [unwired: 1 in]
            n281 = Or(x="Stop z scan", y=w725) -> (x .or. y?=w723:bool)
            n282 = local write "Max vs z"(w734) -> ()
            n283 = Select(t="Action: Find Best Zpos", s=w723, f=w730) -> (s? t:f=w728:string)
          }
        }
        n284 = call <vilib>:"Add State(s) to Queue__jki_lib_state_machine.vi"("State(s) in Front (\"\")"=w688, "State(s) in (\"\")"=w679) -> ("States Out"=w691:string)  [unwired: 13 in]
      }
      frame "Action: Find Best Zpos" {
        n285 = Unbundle By Name(w752) -> ("Hexapod zscan data.Hexapod zscan positions"=w746:dbl[], "Hexapod zscan data.Hexapod zscan diagnostic"=w745:dbl[], "Diagnostic type"=w747:string)
        n286 = case shown="\"Max counts\", Default" w747 {
          tunnel: w745 -> [w758 w761]
          tunnel: [w757 w760] -> w749
          tunnel: [w756 w759] -> w748
          frame "Max counts", Default {
            n287 = Array Max & Min(array=w758) -> (max value=w756:dbl, max index (indices)=w757:i32)  [unwired: 2 out]
          }
          frame "w0 Y" {
            n288 = Array Max & Min(array=w761) -> (min value=w759:dbl, min index (indices)=w760:i32)  [unwired: 2 out]
          }
        }
        "Zpos and w0 Y 2" <- w748
        n289 = Bundle("Hexapod zscan positions"=w746, "Hexapod zscan diagnostic"=w745) -> (→"Max vs z":T6)  [unwired: 1 in]
        n290 = local write "tab"(T9."Z scan" ("tab")) -> ()
        n291 = Index Array(array=w746, index=w749) -> (element=w742:dbl)
        "Zpos and w0 Y" <- w742
        n292 = local write "Central position of z scan"(w742) -> ()
        n293 = Bundle By Name(cluster=w752, "Hexapod zscan data.Best Zpos"=w742) -> (w751:T13)
        n294 = call <vilib>:"Add State(s) to Queue__jki_lib_state_machine.vi"("State(s) in Front (\"\")"="Action: Move>> Best Zpos\nMacro: Alignment", "State(s) in (\"\")"=w755) -> ("States Out"=w754:string)  [unwired: 13 in]
      }
      frame "Action: Send Response" {
        n295 = Unbundle By Name(w772) -> ("NetworkConnection out"=w775:refnum<class "NetworkConnection.lvclass">, "Messages"=w769:i32, "Timer.T1"=w764:i32, "Alignment attempts"=→"Waveform Chart 4":i32)
        "Message count" <- w769
        n296 = Bundle By Name(cluster="Aligned message", "Msg Id"=w769) -> (w770:T4)
        n297 = Increment(x=w769) -> (x+1=w768:i32)
        n298 = call <vilib>:"WriteMessage.vi"("Timeout(ms)"=500, "error in (no error)"=w776, "Message"=w770, "NetworkConnection in"=w775) -> ("error out"=w767:errorcluster, "NetworkConnection out"=w774:refnum<class "NetworkConnection.lvclass">)  [unwired: 4 in, 2 out]
        n299 = call <userlib>:"Tick Count (ms)__ogtk.vi"("error in (no error)"=w767) -> ("error out"=w766:errorcluster, "millisecond timer value"=w765:u32)  [unwired: 9 in]
        n300 = Subtract(x=w765, y=w764) -> (x-y=→"Alignment time" →"Waveform Chart 3":u32)
        n301 = Bundle By Name(cluster=w772, "NetworkConnection out"=w774, "Messages"=w768, "Timer.T2"=w765) -> (w773:T13)
        n302 = call <vilib>:"Add State(s) to Queue__jki_lib_state_machine.vi"("State(s) in (\"\")"=w779) -> ("States Out"=w778:string)  [unwired: 14 in]
      }
    }
  }
  n303 = disable-structure shown="Disabled" {
    frame Disabled {
      n304 = Unbundle By Name() -> ()  [unwired: 1 in, 1 out]
      n305 = Bundle By Name("Alignment attempts"=0) -> ()  [unwired: 1 in, 1 out]
      n306 = Greater?(y=10) -> (x=w781:i32)  [unwired: 1 out]
    }
    frame Enabled {
    }
  }
